vi "V1.2_UI.vi"() -> ()   [LabVIEW 2018]
uses:
  <vilib>/MakerHub/LINX/Private/Type Defs/LINX Ref.ctl
  <vilib>/MakerHub/LINX/Private/Type Defs/Platform.ctl
  <vilib>/MakerHub/LINX/Private/Type Defs/Interface.ctl
  <vilib>/MakerHub/LINX/Private/Device/Type Defs/LINX Device Config.ctl
  <vilib>/MakerHub/LINX/Private/Device/Type Defs/TCP Config.ctl
  <vilib>/MakerHub/LINX/Private/Device/Type Defs/Channels.ctl
  C:/Users/e14user/Documents/LabVIEW software/GitRepo/lib/tiff/LVTiffWriter/BitMiracle.LibTiff.NET.dll
  lib/tiff/LVTiffWriter/BitMiracle.LibTiff.NET.dll
  <vilib>/MakerHub/LINX/Public/Utilities/Open Serial.vi
  lib/Olympus IX BX Series/Olympus IX BX Series.lvlib
  <vilib>/MakerHub/LINX/LMH-LINX.lvlib
  lib/SOLA/LabVIEW 2015 Library (32bit)/LumencorDLL32/LumencorDLL32.lvlib
  lib/ANDOR/Andor SDK/AndorSDK.lvlib
  lib/ANDOR/OwnVIs/AndorOWN.lvlib
  lib/TANGO Stage/TangoOWN.lvlib
  <userlib>/Tango_DLL/Tango_DLL.lvlib
  lib/ARDUINO/VIs/Arduino.lvlib
  lib/Config/Config.lvlib
  lib/tiff/LVTiffWriter/LVTiffWriter.lvlib
  lib/ContinuousLoop/ContinousLoop.lvlib
  <vilib>/vision/NI_Vision_Development_Module.lvlib
  lib/Calib/Calibration.lvlib
  <vilib>/MakerHub/LINX/Private/Device/Device.lvlib
panel:
  out "CalibRemainingTime":dbl caption="Rem. Time" format="%<%H:%M:%S%2u>t"
  in  "CalibRestart":bool
  in  "Calib Feed Cycles":i32=3 caption="Feed Cycles"
  in  "Calib Pump Cycles":i32=10 caption="Pump Cycles"
  in  "AndorHistRange":cluster{"Minimum":sgl, "Maximum":sgl}={"Minimum"=0.0, "Maximum"=65535.0} caption="Range" {"Maximum" min=217 max=912 scale=217.0..912.0; "Minimum" min=217 max=912 scale=217.0..912.0}
  out "ANDORHistMaxValue":dbl
  out "ANDORHistMinValue":dbl
  out "ValveConnSuccess":bool
  in  "ValvePort":refnum<visa-resource-name>="COM7" caption="Valve Controller"
  out "IX81ConnSuccess":bool caption="IX81 Conn Success"
  in  "IX 81 Port":refnum<visa-resource-name>="IX2-UCB"
  out "SOLAConnSuccess":bool
  in  "SOLAPort":refnum<visa-resource-name>="COM5" caption="SOLA COM Port"
  in  "PosListClearLast":bool
  in  "PosListCapture":bool caption="Save Pos"
  out "Program Timing Offset":dbl
  in  "IX81SettingsSave":bool caption="Save Microscope Settings"
  in  "ProgramRun":bool
  out "CalibTiffHandle":refnum<k24> caption="TiffHandle"
  out "CalibInstructions":string="First, capture a blank by adjusting the microscope for a brightfield image of the empty channel. Adjust exposure, objective and filters accordingly. Test it using single images!" caption="Instructions"
  in  "ProgramCreate":bool
  in  "IX81SettingsClear":bool caption="Clear Microscope Settings"
  in  "IX81SettingsAppend":bool caption="Append Current Settings"
  out "CalibImgPath":path caption="Location of Calibration Image File"
  in  "CalibPumpCycleRefreshRatio":dbl=0.01 caption="singlePumpCycleRefreshRatio"
  in  "IX81Settings":i32(listbox) caption="Microscope Settings"
  in  "CalibStart":bool
  out "ProgramProgress":u8(slide) scale=0.0..100.0
  in  "ProgramStop":bool
  out "error out":errorcluster
  out "ProgramXML":string caption="XML"
  out "LINX Resource":T1={"IO"=enum."Remote", "Interface"=enum."TCP", "LINX Device Config"={"Interface"=enum."Serial", "COM Port"="COM13", "TCP Configuration"={"IP Address"="", "Port"=0}, "Device Family"=1, "Device ID"=1, "Device Name"="myRIO-1900", "TCP Ref"=refnum, "Channels"={"DI"=[0, 1, 2, 3, 4, 5, 6, 7, 8, 9, 10, 11, 12, 13, 14, 15, 16, 17, 18, 19, 20, 21, 22, 23, 24, 25, 26, 27, 28, 29, 30, 31, 32, 33, 34, 35, 36, 37, 38, 39, 40, 41, 42, 43, 44, 45, 46], "DO"=[0, 1, 2, 3, 4, 5, 6, 7, 8, 9, 10, 11, 12, 13, 14, 15, 16, 17, 18, 19, 20, 21, 22, 23, 24, 25, 26, 27, 28, 29, 30, 31, 32, 33, 34, 35, 36, 37, 38, 39, 40, 41, 42, 43, 44, 45, 46], "AI"=[0, 1, 2, 3, 4, 5, 6, 7, 8, 9, 10, 11], "AO"=[], "PWM"=[3, 5, 6, 9, 10], "QE"=[], "UART"=[0, 1], "I2C 2"=[0], "SPI"=[0], "CAN"=[], "Servo"=[], "AI Ref (V)"=0.0, "AI Resolution (Bits)"=0, "AO Ref (V)"=0.0, "AO Resolution (Bits)"=0}}}
  out "elements":cluster{"Button":string, "Value":dbl}[](array[cluster])
  out "ANDORAcqErrors":cluster{i32, string}[](array[cluster]) caption="Acqisition Error Array"
  out "ProgramKeysPressed":T7(array[ring]) caption="keys pressed"
  out "TANGOConnError":i32 caption="Tango Connection\n Error"
  in  "PosListSaveXML":bool caption="Save Pos List"
  in  "PosList":i32[](listbox) caption="Position List"
  in  "ValveOpenAll":bool caption="Open all"
  in  "ValveCloseAll":bool caption="Close all"
  in  "C8":bool
  in  "C7":bool
  in  "C6":bool
  in  "C5":bool
  in  "C4":bool
  in  "C3":bool
  in  "C2":bool
  in  "C1":bool
  in  "B8":bool
  in  "B7":bool
  in  "B6":bool
  in  "B5":bool
  in  "B4":bool
  in  "B3":bool
  in  "B2":bool
  in  "B1":bool
  in  "A8":bool
  in  "A7":bool
  in  "A6":bool
  in  "A5":bool
  in  "A4":bool
  in  "A3":bool
  in  "A2":bool
  in  "A1":bool
  in  "ANDORColormap":u16(ring) caption="Colormap" items=["Grey", "Hot"]
  in  "ANDORImgFormat":u16(ring)=6 caption="Format"
  in  "ANDORImgPath":path caption="Path"
  in  "ANDORImgName":string="TestIMG" caption="Image Name"
  in  "ANDORImgSave":bool caption="ANDORSave Image"
  out "SOLA":u32
  out "TANGO":i32
  out "ANDORExposureMeas":sgl caption="Exposure" format="%#_g s"
  out "ANDORAccum":sgl caption="Accum."
  out "ANDORKinetic":sgl caption="Kinetic"
  out "ANDORTemperature":sgl caption="Temperature" format="%.2f °C"
  out "ANDORImage":T8(plugin-control)
  in  "IX81Filter":u16(ring)=6 caption="Filter:" items=["UV ", "CFP", "YFP", "RFP", "Cy5", "GFP", "Bright Field"]
  in  "IX81Prism":u16(ring)=1 caption="Prism" items=["Bi", "Side"]
  in  "IX81Objective":enum16{"x 4", "x 10", "x 20", "x 40", "x 100"}(ring) caption="Objective"
  in  "IX81Focus":dbl caption="Focus [µm]" format="%.3f"
  out "IX81LimitTop":dbl caption="Upper Limit"
  out "IX81LimitBottom":dbl caption="Lower Limit"
  in  "IX81Intensity":dbl(slide) caption="Intensity [%]" scale=0.0..100.0 scale format="%.1f"
  in  "ANDORExposure":sgl=50.0 caption="Exposure" format="%#_g ms"
  in  "ANDORLive":bool
  in  "ANDORImgSingle":bool
  in  "TANGODown":bool
  in  "TANGOLeft":bool caption="Left"
  in  "TANGOUp":bool
  in  "TANGORight":bool
  in  "ProgramSingleMultiring":bool=TRUE caption="Which chip are you using?"
  in  "ValveFeedRingAll":bool caption="Actuate all Rings at once?"
  in  "ValveFlushReagent":u16 caption="Flush\nReagent"
  in  "ValveFlushOn":bool caption="Flush"
  in  "ValvePumpCycles":dbl=10.0 caption="Pump Cycles"
  in  "ValvePumpFrequency":dbl=10.0 caption="Frequency" format="%#_3f"
  in  "ValvePumpOn":bool caption="Pump On"
  in  "ValveFeedOn":bool caption="Feed On"
  in  "ValveFeedCycles":i32=10 caption="Feed Cycles"
  in  "ValveFeedReagent":u16=2 caption="Feed\nReagent"
  in  "ValveFeedRing":u16 caption="Ring"
  in  "TANGOCalibrate":bool caption="Calibrate"
  out "TANGOyLimits":dbl[](array[numeric]) caption="Y Limits [µm]" format="%#_12f"
  out "TANGOxLimits":dbl[](array[numeric]) caption="X Limits [µm]" format="%#_10f"
  in  "TANGOStep":dbl=100.0 caption="Step Width [µm]" min=0.0 format="%#_6f"
  out "TANGOPosition":dbl[](array[numeric]) caption="Position [µm]" format="%#_12f"
  out "TANGOConnSuccess":bool
  in  "TANGOPort":refnum<visa-resource-name>="COM4" caption="TANGO COM Port"
  out "ProgramStatusInfo":string caption="String"
  # "Calibration of a Microfluidic Pump"
  # "Execute Continuous Progam"
  # "Error Messages"
  # "More information below"
  # "Various Error and Status Messages"
  # "Position List"
  # "Manual Valves"
  # "Save Image"
  # "OneRing"
  # "Multiring"
  # "Microfluidics"
  # "Valve Functions"
  # "min"
  # "max"
  # "min"
  # "max"
  # "X"
  # "Y"
  # "Stage"
  # "Initialization"
  # "Microscope"
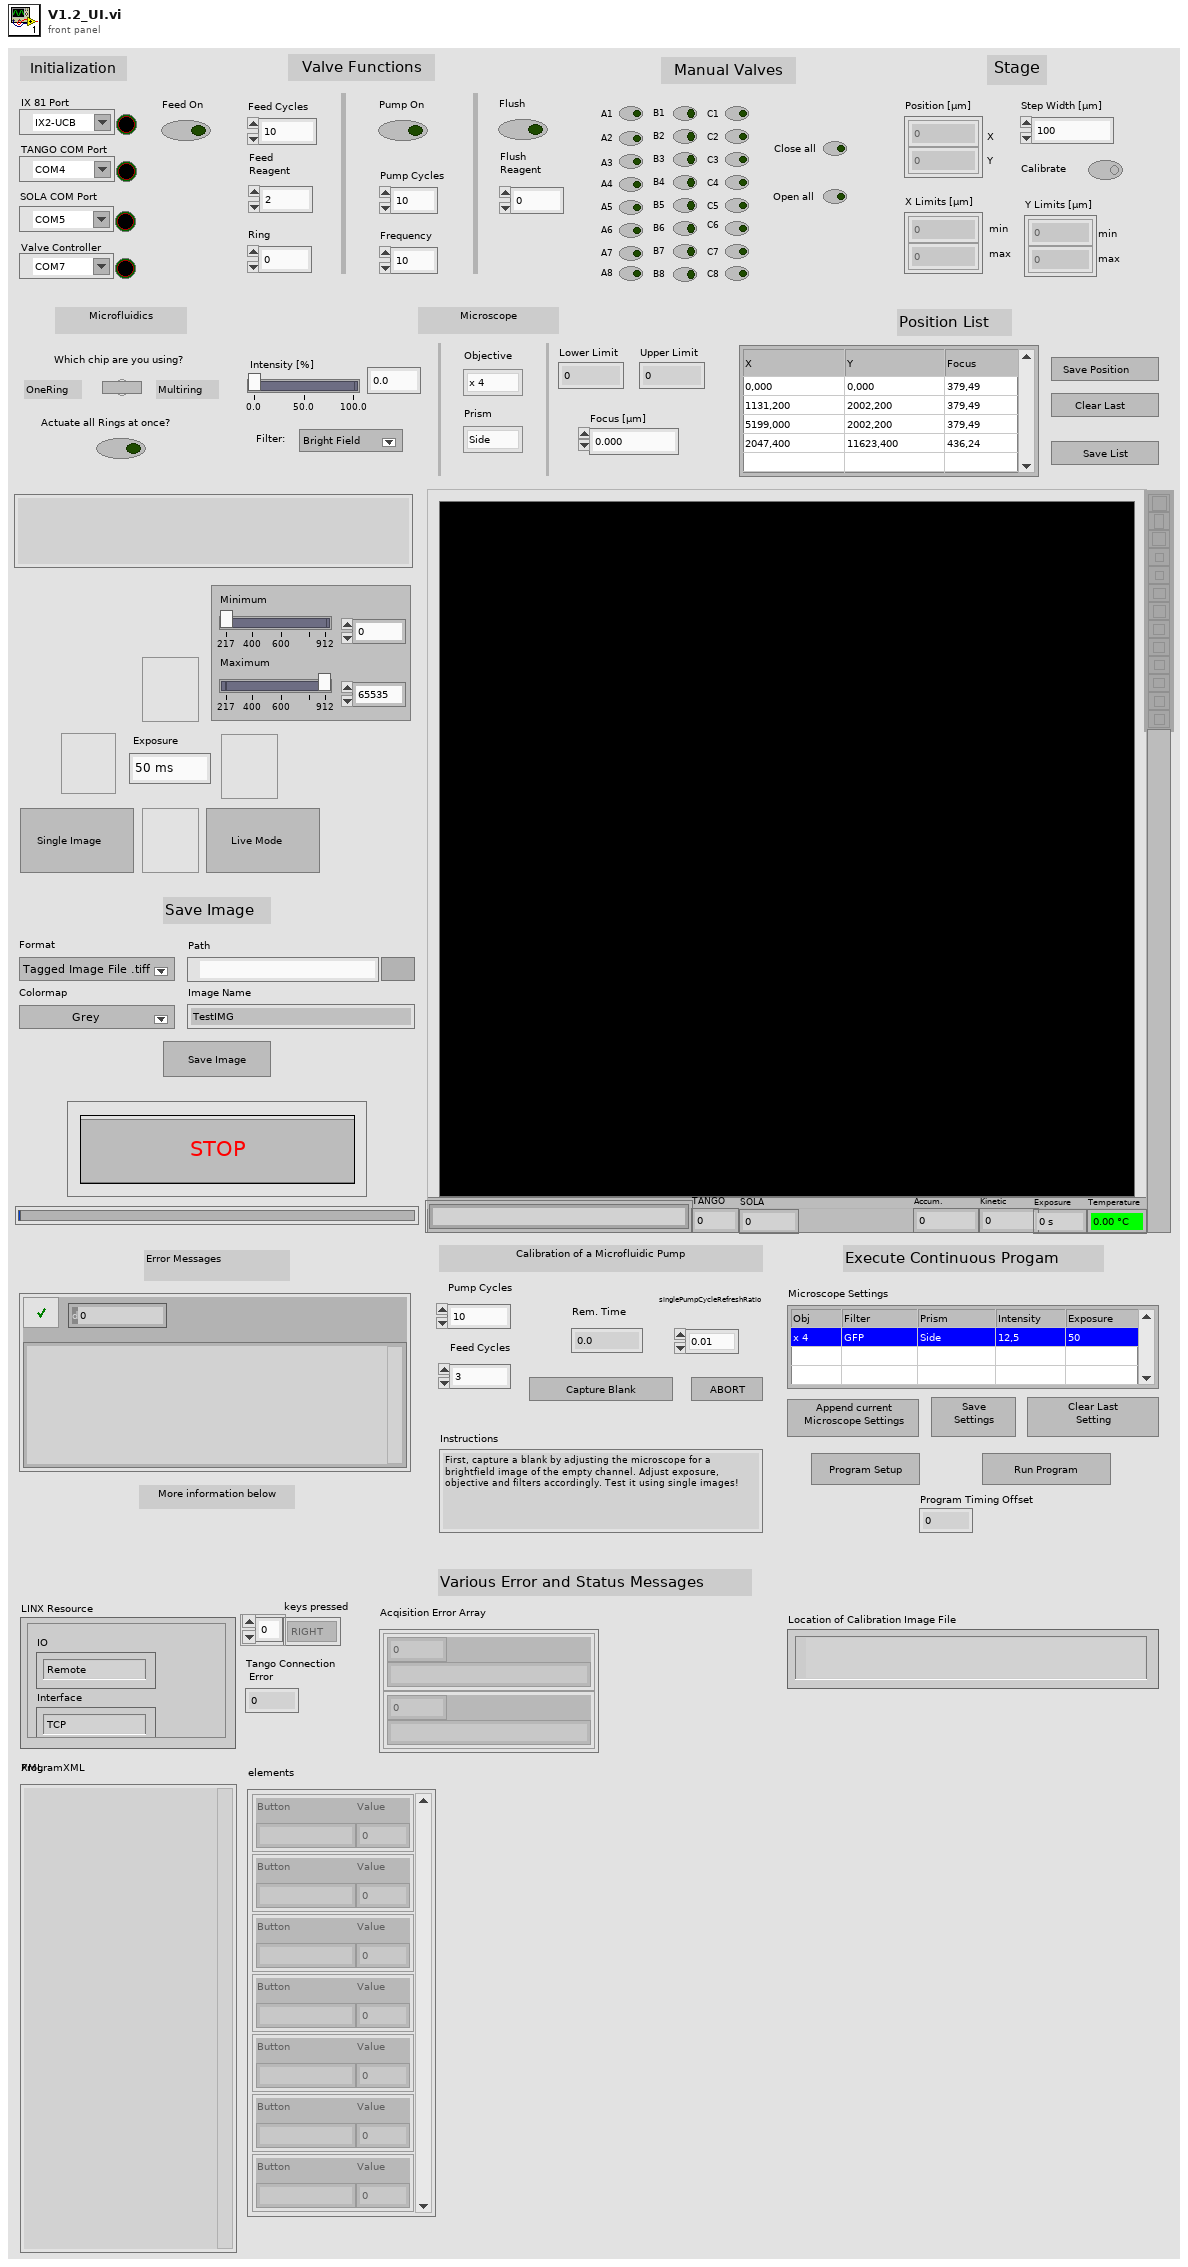
[diagram p1: front panel]
types:
  T1 = typedef "LMH-LINX.lvlib/LINX Ref.ctl" = cluster{"IO":T2, "Interface":T3, "LINX Device Config":T4}
  T2 = typedef "LMH-LINX.lvlib/Platform.ctl" = enum16{"Remote", "Local"}
  T3 = typedef "LMH-LINX.lvlib/Interface.ctl" = enum16{"Serial", "TCP"}
  T4 = typedef "LMH-LINX.lvlib/Device.lvlib/LINX Device Config.ctl" = cluster{"Interface":T3, "COM Port":refnum<visa-resource-name>, "TCP Configuration":T5, "Device Family":u8, "Device ID":u8, "Device Name":string, "TCP Ref":refnum<k5>, "Channels":T6}
  T5 = typedef "LMH-LINX.lvlib/Device.lvlib/TCP Config.ctl" = cluster{"IP Address":string, "Port":u16}
  T6 = typedef "LMH-LINX.lvlib/Channels.ctl" = cluster{"DI":u8[], "DO":u8[], "AI":u8[], "AO":u8[], "PWM":u8[], "QE":u8[], "UART":u8[], "I2C 2":u8[], "SPI":u8[], "CAN":u8[], "Servo":u8[], "AI Ref (V)":dbl, "AI Resolution (Bits)":u8, "AO Ref (V)":dbl, "AO Resolution (Bits)":u8}
  T7 = enum16{"0", "1", "2", "3", "4", "5", "6", "7", "8", "9", "A", "B", "C", "D", "E", "F", "G", "H", "I", "J", "K", "L", "M", "N", "O", "P", "Q", "R", "S", "T", "U", "V", "W", "X", "Y", "Z", "F1", "F2", "F3", "F4", "F5", "F6", "F7", "F8", "F9", "F10", "F11", "F12", "F13", "F14", "F15", "ADD", "BACK", "BACKSLASH", "CAPITAL", "COMMA", "DECIMAL", "DELETE", "DIVIDE", "DOWN", "END", "EQUALS", "ESCAPE", "GRAVE (`)", "HOME", "INSERT", "LBRACKET", "LCONTROL", "LEFT", "L ALT", "LSHIFT", "LWIN", "MINUS", "MULTIPLY", "NEXT", "NUMLOCK", "NUMPAD_0", "NUMPAD_1", "NUMPAD_2", "NUMPAD_3", "NUMPAD_4", "NUMPAD_5", "NUMPAD_6", "NUMPAD_7", "NUMPAD_8", "NUMPAD_9", "PAUSE", "PERIOD", "PRIOR (PG UP)", "RBRACKET", "RCONTROL", "RETURN", "RIGHT", "R ALT", "RSHIFT", "RWIN", "SCROLL", "SEMICOLON", "SLASH", "SPACE", "SUBTRACT", "TAB", "UP", "ENTER (num pad)", "' (quote)"}[]
  T8 = typedef "IMAQ Image.ctl" = refnum<image>
  T9 = enum8{"Enabled", "Disabled", "Disabled and Grayed Out"}
  T10 = enum32{"Linear", "Log", "Exp", "Square", "Square root", "Power X", "Power 1/X"}
  T11 = enum16{"open", "replace", "create", "open or create", "replace or create", "replace or create with confirmation"}
  T12 = typedef "Image Type" = u32
  T13 = cluster{"histogram":u32[], "Minimal Value":sgl, "Maximal Value":sgl, "Starting Value":sgl, "Interval Width":sgl, "Mean Value":sgl, "Standard  Variation":sgl, "Area (pixels)":i32}
  T14 = cluster{string, "NewVal":enum16{"x 4", "x 10", "x 20", "x 40", "x 100"}}
  T15 = cluster{"Objective":i32, "Filter":string, "Prism":string, "Intensity":dbl, "Exposure":i32}[]
  T16 = cluster{"Step Name":string, "Time":dbl, "Param 1":dbl, "Param 2":i32}
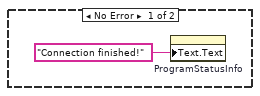
[diagram p2: hidden frame]
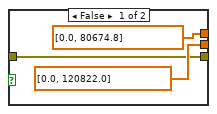
[diagram p3: hidden frame]
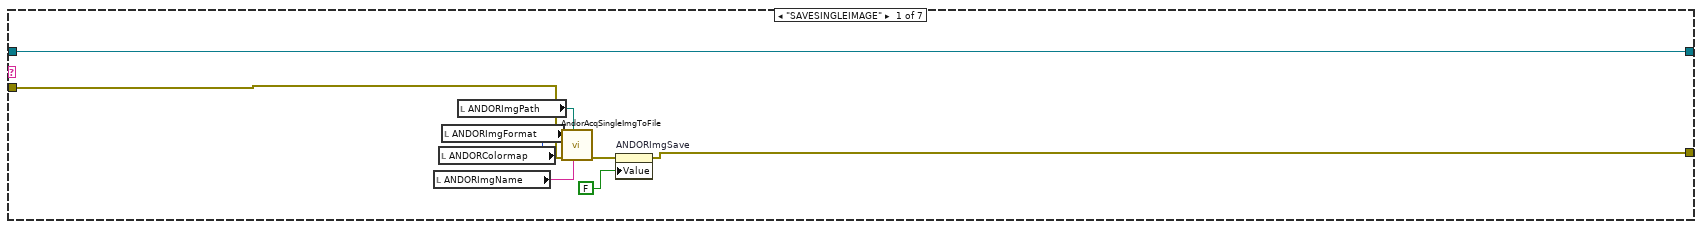
[diagram p4: hidden frame]
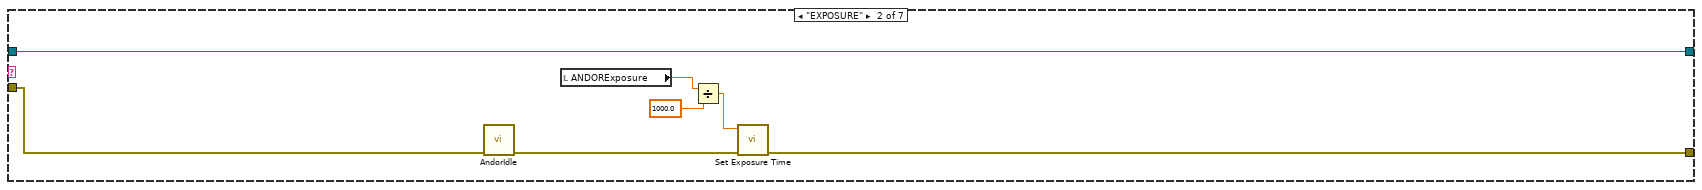
[diagram p5: hidden frame]
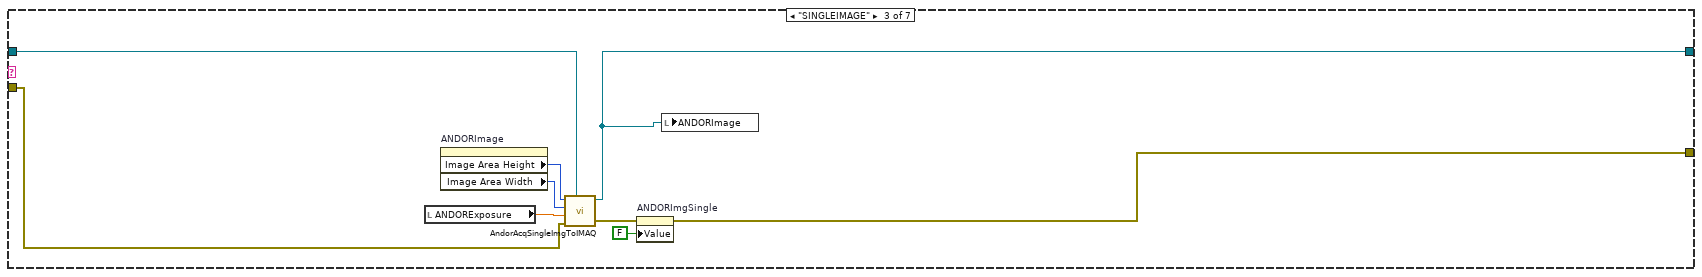
[diagram p6: hidden frame]
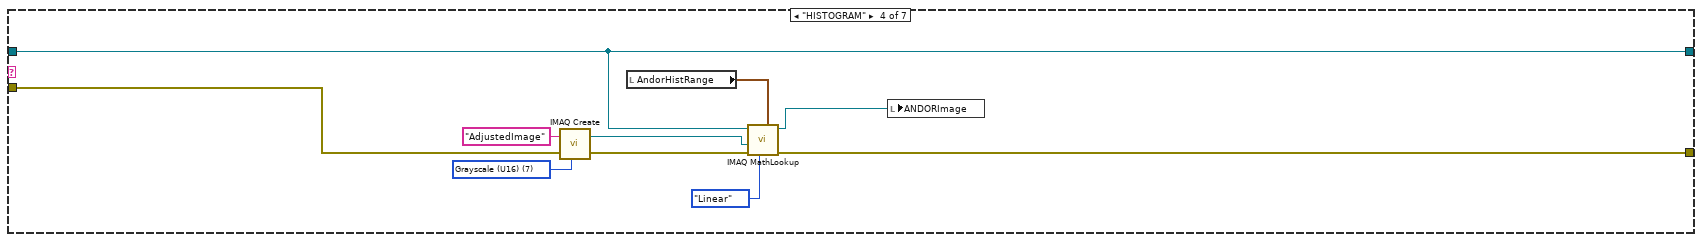
[diagram p7: hidden frame]
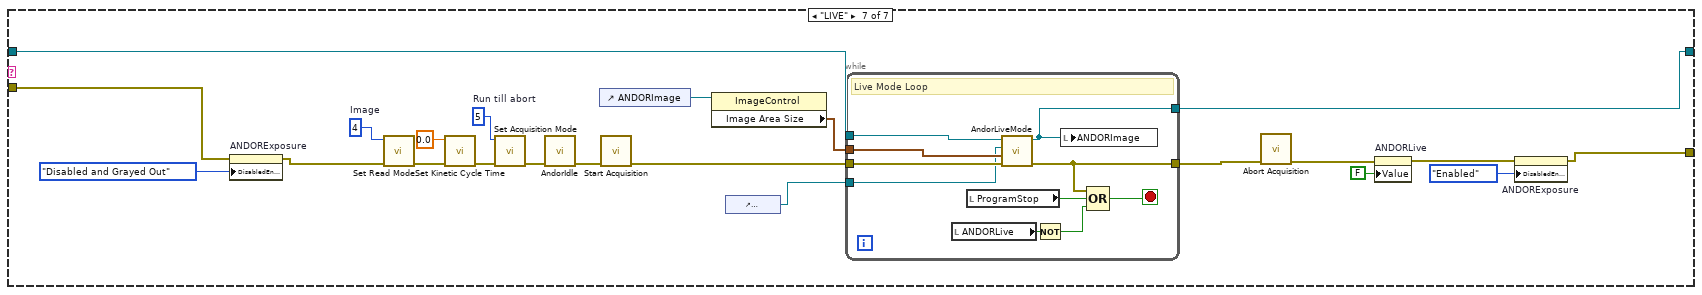
[diagram p9: hidden frame]
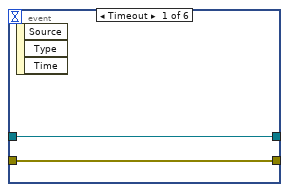
[diagram p10: hidden frame]
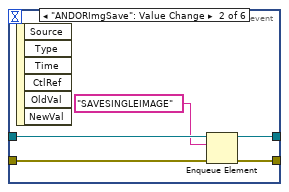
[diagram p11: hidden frame]
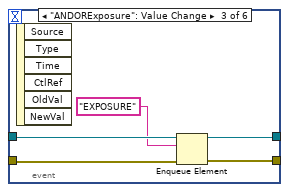
[diagram p12: hidden frame]
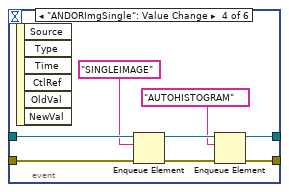
[diagram p13: hidden frame]
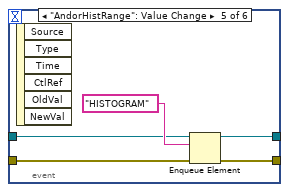
[diagram p14: hidden frame]
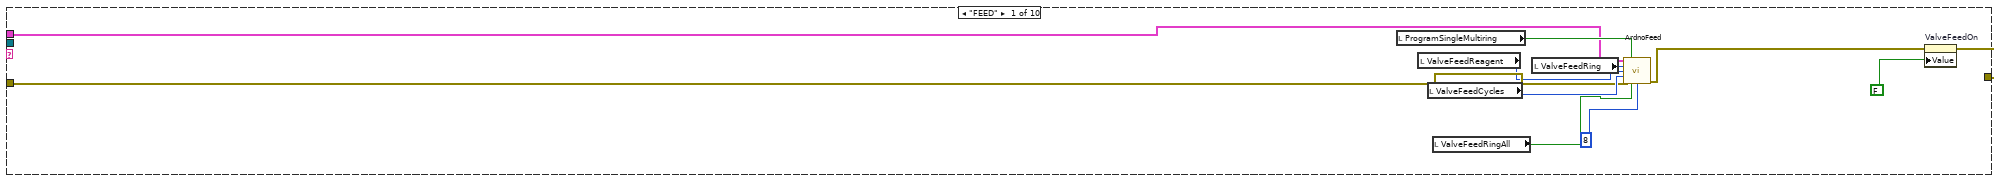
[diagram p16: hidden frame]
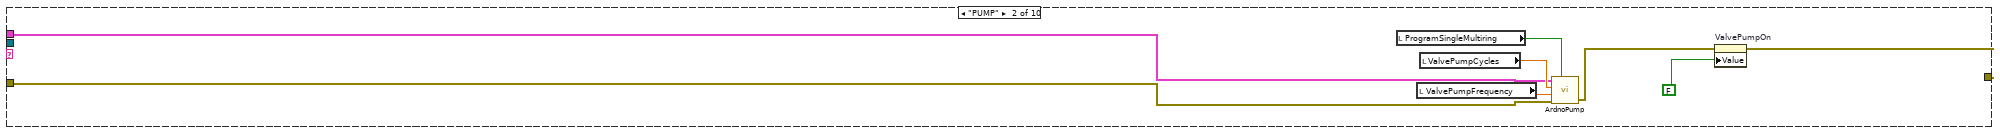
[diagram p17: hidden frame]
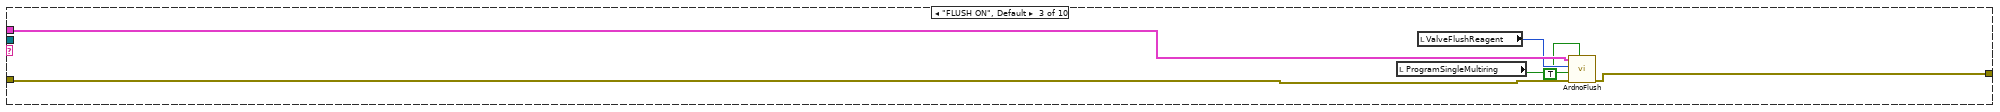
[diagram p18: hidden frame]
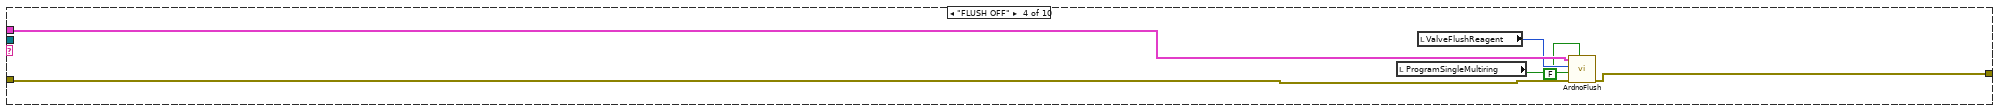
[diagram p19: hidden frame]
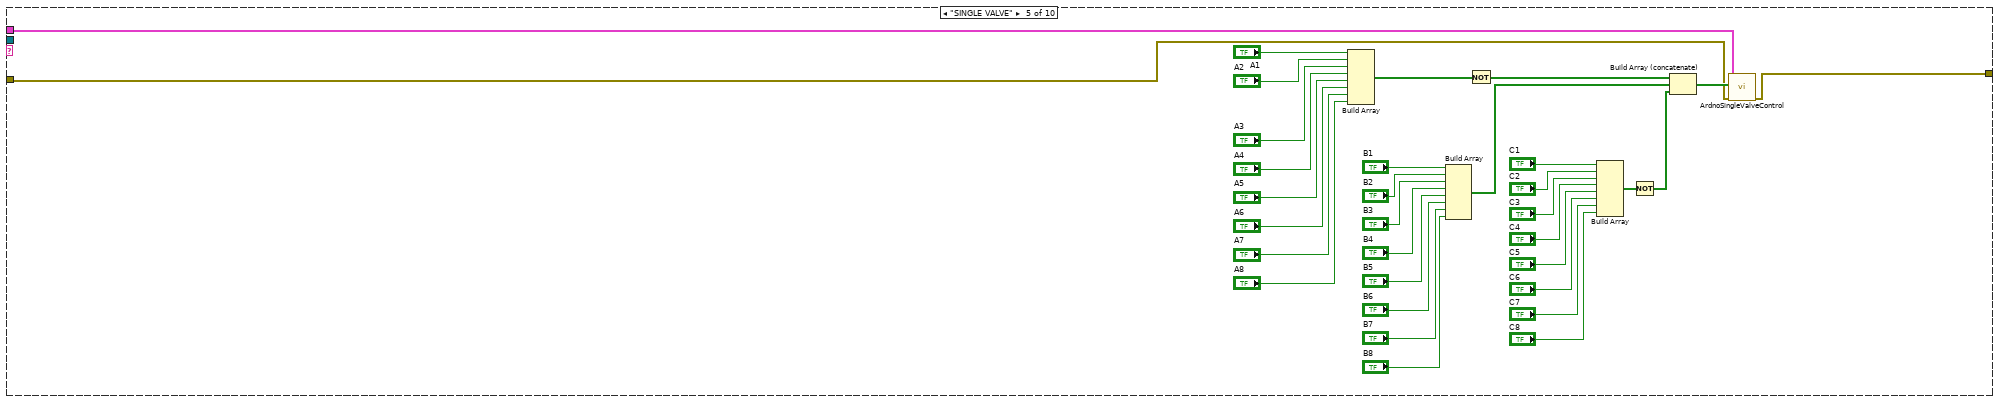
[diagram p20: hidden frame]
diagram:
  n1 = flat-sequence {
    tunnel: [w32] -> w9
    tunnel: [w31] -> w8
    tunnel: [w30] -> w7
    tunnel: [w29] -> w6
    tunnel: [w28] -> w5
    tunnel: [w80] -> w19
    tunnel: w9 -> [w73]
    tunnel: w8 -> [w72]
    tunnel: w7 -> [w71]
    tunnel: w6 -> [w65]
    tunnel: w5 -> [w70]
    tunnel: [w69] -> w4
    tunnel: [w68] -> w3
    tunnel: [w64] -> w2
    tunnel: [w67] -> w1
    tunnel: [w109] -> w20
    tunnel: w19 -> [w110]
    tunnel: w4 -> [w108]
    tunnel: w3 -> [w107]
    tunnel: w2 -> [w106]
    tunnel: w1 -> [w105]
    tunnel: w20 -> [w1609]
    tunnel: [w1603] -> w12
    frame #0 {
      w21 = cluster{u32, u32}[] [{16711680, 0}, {65280, 0}, {6710886, 0}, {6710886, 0}] ("Colors [4]")
      # "Connection String"
      n2 = local write "ProgramStatusInfo"("Connecting..." ("Info")) -> ()
      n3 = property on="CalibStart" class="Bool (strict)"("BoolText.Text"="Capture Blank" ("Boolean Text.Text")) -> ()  [unwired: 2 in, 2 out]
      n4 = property on="Pane" class="Pane"() -> ("Controls[]"=w23:refnum<vi>[])  [unwired: 2 in, 2 out]
      n5 = for {
        tunnel: w23 -> [w27] mode=indexing
        tunnel: T9."Enabled" ("Disabled") -> [w26]
        n6 = property class="Ctl"(reference=w27, "DisabledEnum"=w26) -> ()  [unwired: 1 in, 2 out]
      }
      n7 = property on="IX81ConnSuccess" class="Bool (strict)"("Colors [4]"=w21) -> ()  [unwired: 2 in, 2 out]
      n8 = property on="TANGOConnSuccess" class="Bool (strict)"("Colors [4]"=w21) -> ()  [unwired: 2 in, 2 out]
      n9 = property on="SOLAConnSuccess" class="Bool (strict)"("Colors [4]"=w21) -> ()  [unwired: 2 in, 2 out]
      n10 = property on="ValveConnSuccess" class="Bool (strict)"("Colors [4]"=w21) -> ()  [unwired: 2 in, 2 out]
    }
    frame #1 {
      w55 = 2  # Device Number (1: Condensor, Objective Lamp,Shutter 2: Z-Motion, Autofocus)
      w58 = 1  # Device Number (1: Condensor, Objective Lamp,Shutter 2: Z-Motion, Autofocus)
      # "Establishing Connections To All Devices"
      n11 = property on="SOLAPort" class="VISAName"() -> ("Text.Text"=w42:string)  [unwired: 2 in, 2 out]
      n12 = Scan From String(format string="COM%d", input string=w42) -> (output 1=w51:i32)  [unwired: 3 in, 3 out]
      n13 = local read "TANGOPort"() -> (w45:refnum<visa-resource-name>)
      n14 = local read "ValvePort"() -> (w53:refnum<visa-resource-name>)
      n15 = Decrement(x=w51) -> (x-1=w50:i32)
      n16 = local read "IX 81 Port"() -> (w54:refnum<visa-resource-name>)
      n17 = call-poly <vilib>:"Open.vi"("Serial Port"=w53) -> ("Error Out"=w29:errorcluster, "LINX Resource"=→"LINX Resource":T1)  [unwired: 8 in, 1 out]
      n18 = call "lm Init.vi"("LETypeStr"="SOLA", "ComPort"=w50) -> ("error out"=w30:errorcluster, "LETypeStr out"=w41:string, "function return"=→"SOLA":u32)  [unwired: 7 in]
      n19 = call "Initialize.vi"("VISA Resource Name"=w54) -> ("VISA Resource Name Out"=w59:refnum<visa-resource-name>, "error out"=w60:errorcluster)  [unwired: 13 in]
      n20 = call "Initialize.vi"("dir"="C:\\Users\\e14user\\Documents\\LabVIEW software\\GitRepo\\lib\\ANDOR\\Libraries") -> ("error out"=w31:errorcluster)  [unwired: 8 in, 2 out]
      n21 = call "TangoConnect.vi"("Tango Com"=w45) -> ("error out"=w32:errorcluster, "success"=w43:bool, "plLSID out"=→"TANGO":i32)  [unwired: 7 in, 1 out]
      n22 = Unbundle By Name(w30) -> ("status"=w39:bool)
      n23 = Unbundle By Name(w29) -> ("status"=w35:bool)
      n24 = call "Login Device.vi"("error in (no error)"=w60, "Device Number (1)"=w58, "VISA Resource Name"=w59) -> ("error out"=w56:errorcluster, "VISA Resource Name Out"=w57:refnum<visa-resource-name>)  [unwired: 7 in]
      n25 = Empty String/Path?(string/path=w41) -> (empty?=w40:bool)
      n26 = local write "TANGOConnSuccess"(w43) -> ()
      n27 = Not(x=w35) -> (.not. x?=w34:bool)
      n28 = Not Or(1:w39, 2:w40) -> (0:w38:bool)
      n29 = call "Login Device.vi"("error in (no error)"=w56, "Device Number (1)"=w55, "VISA Resource Name"=w57) -> ("error out"=w28:errorcluster)  [unwired: 7 in, 1 out]
      n30 = local write "ValveConnSuccess"(w34) -> ()
      n31 = local write "SOLAConnSuccess"(w38) -> ()
      n32 = Unbundle By Name(w28) -> ("status"=w37:bool)
      n33 = Not(x=w37) -> (.not. x?=w33:bool)
      n34 = local write "IX81ConnSuccess"(w33) -> ()
      n35 = Merge Errors(w28, w29, w30, w32, w31) -> (w47:errorcluster)
      n36 = case shown="Error" w47 {
        frame No Error {
          n37 = property on="ProgramStatusInfo" class="Str"("Text.Text"="Connection finished!") -> ()  [unwired: 2 in, 2 out]
        }
        frame Error {
          n38 = property on="ProgramStatusInfo" class="Str"("Text.Text"="Connection did not work!\nTry restarting the respective device.") -> ()  [unwired: 2 in, 2 out]
        }
      }
    }
    frame #2 {
      # "Initializing Devices With (Config File)"
      n39 = local read "LINX Resource"() -> (w66:T1)
      n40 = local read "IX 81 Port"() -> (w94:refnum<visa-resource-name>)
      n41 = local read "ANDORExposure"() -> (w85:sgl)
      n42 = local read "TANGOCalibrate"() -> (w89:bool)
      n43 = local write "IX81LimitTop"(3000000.0 ("default (0 I32)")) -> ()
      n44 = local write "IX81LimitBottom"(10.0 ("Upper Limit")) -> ()
      n45 = call "AndorInitCamera.vi"("error in (no error)"=w72, "Exposure"=w85) -> ("error out"=w69:errorcluster, "accumulate out"=w82:sgl, "exposure out"=w83:sgl, "temperature out"=w86:sgl, "kinetic out"=w84:sgl)  [unwired: 5 in]
      n46 = call "lm Color Enable.vi"("error in (no error)"=w71, "str_State"="ON", "str_Color"="WHITE") -> ("error out"=w75:errorcluster, "str_Color out"=w76:string)  [unwired: 6 in, 1 out]
      n47 = call "OlympusInitialize.vi"("error in (no error)"=w70, "IX81 in"=w94) -> ("error out"=w67:errorcluster, "Objective"=w92:i32, "Focus Position"=w81:dbl, "Prism Position (0: Bi)"=w78:enum16{"Bi", "Side"}, "Filter"=w93:i32, "Intensity [%]"=w79:dbl)  [unwired: 4 in]
      n48 = case shown="True" w89 {
        tunnel: [w97 w104] -> w68
        tunnel: w73 -> [w97 w100]
        tunnel: [dbl[] [0.0, 80674.8] ("Y Limits") w103] -> w87
        tunnel: [dbl[] [0.0, 120822.0] ("X Limits") w102] -> w88
        frame False {
        }
        frame True {
          n49 = local read "TANGO"() -> (w101:i32)
          n50 = call "TangoCalibrate.vi"("error in (no error)"=w100, "plLSID in"=w101) -> ("error out"=w104:errorcluster, "X Limits"=w102:dbl[], "Y Limits"=w103:dbl[])  [unwired: 7 in]
        }
      }
      n51 = call "ArdnoAllValvesOpened.vi"("Single/\nMultiring?"=TRUE ("Single/\nMultiring?"), "error in (no error)"=w65, "LINX Resource"=w66) -> ("error out"=w64:errorcluster)  [unwired: 7 in, 1 out]
      n52 = local write "ANDORKinetic"(w84) -> ()
      n53 = local write "ANDORTemperature"(w86) -> ()
      n54 = local write "ANDORExposureMeas"(w83) -> ()
      n55 = local write "ANDORAccum"(w82) -> ()
      n56 = call "lm Color Level.vi"("error in (no error)"=w75, "str_Level"="0", "str_Color"=w76) -> ("error out"=w74:errorcluster)  [unwired: 6 in, 2 out]
      n57 = local write "TANGOyLimits"(w87) -> ()
      n58 = local write "TANGOxLimits"(w88) -> ()
      n59 = local write "IX81Intensity"(w79) -> ()
      n60 = local write "IX81Prism"(w78) -> ()
      n61 = local write "IX81Focus"(w81) -> ()
      n62 = local write "IX81Objective"(w92) -> ()
      n63 = local write "IX81Filter"(w93) -> ()
      n64 = Merge Errors(w67, w64, w74, w68, w69) -> (w80:errorcluster)
    }
    frame #3 {
      n65 = while {
        shift-right: [w117] -> w109
        shift-left: w110 -> [w116]
        tunnel: w108 -> [w114]
        tunnel: w107 -> [w113]
        tunnel: w106 -> [w112]
        tunnel: w105 -> [w111]
        stop <- w115 stop-if-true
        n66 = stacked-sequence {
          tunnel: [w122 _] -> w117
          tunnel: w116 -> [_ _]
          tunnel: w114 -> [w121 _]
          tunnel: w113 -> [w120 _]
          tunnel: w112 -> [w119 _]
          tunnel: w111 -> [w118 _]
          frame #0 {
            n67 = while {
              tunnel: w120 -> [w151]
              tunnel: w119 -> [w150]
              tunnel: w118 -> [w149]
              shift-right: [w123] -> w122
              shift-left: w121 -> [w152]
              stop <- w126 stop-if-true
              w136 = 1122  # Clear Queue Invalid Error
              w162 = T12 7 items=["Grayscale (U8)", "Grayscale (I16)", "Grayscale (SGL)", "Complex (CSG)", "RGB (U32)", "HSL (U32)", "RGB (U64)", "Grayscale (U16)"] ("Image Type")
              w194 = ""  # Button
              n68 = call "IMAQ Create"("Image Name"="RawImage", "Image Type"=w162) -> ("New Image"=w163:T8, "error out"=w145:errorcluster)  [unwired: 3 in]
              n69 = local read "TANGO"() -> (w205:i32)
              n70 = local read "LINX Resource"() -> (w201:T1)
              n71 = Obtain Queue(name (unnamed)="CameraQueue", element data type="", error in (no error)=w152) -> (queue out=w185:refnum<queue>, error out=w184:errorcluster)  [unwired: 2 in, 1 out]
              n72 = Obtain Queue(name (unnamed)="StageCTRL", element data type="" ("Button"), error in (no error)=w151) -> (queue out=w197:refnum<queue>, error out=w177:errorcluster)  [unwired: 2 in, 1 out]
              n73 = local read "IX 81 Port"() -> (w167:refnum<visa-resource-name>)
              n74 = Obtain Queue(name (unnamed)="FluidCTRL", element data type=w194, error in (no error)=w150) -> (queue out=w200:refnum<queue>, error out=w199:errorcluster)  [unwired: 2 in, 1 out]
              n75 = Obtain Queue(name (unnamed)="MicroscopeCTRL", element data type=cluster{"Button":string, "Value":dbl} {"Button"="", "Value"=0.0}, error in (no error)=w149) -> (queue out=w196:refnum<queue>, error out=w148:errorcluster)  [unwired: 2 in, 1 out]
              n76 = Merge Errors(w145, w184) -> (w146:errorcluster)
              n77 = while {
                tunnel: 5 -> [w297]
                tunnel: w185 -> [w292]
                tunnel: [w290] -> w156
                tunnel: w184 -> [w291]
                tunnel: [w289] -> w154
                stop <- w294 stop-if-true
                # "ANDOR CAMERA MEssage Loop"
                n78 = event shown="[5] \"ANDORLive\": Value Change" {
                  selector: _ -> [_ _ _ _ _ _]
                  dyn-events: _ -> [_ _ _ _ _ _]
                  timeout: w297 -> [_ _ _ _ _ _]
                  tunnel: w292 -> [w299 w304 w309 w317 w321 w329]
                  tunnel: w291 -> [w298 w303 w308 w316 w320 w330]
                  tunnel: [w298 w300 w306 w311 w319 w323] -> w289
                  tunnel: [w299 w301 w307 w313 w318 w324] -> w290
                  event Timeout {
                    n79 = event-data() -> ()  [unwired: 1 in, 3 out]
                  }
                  event "ANDORImgSave": Value Change {
                    n80 = event-data() -> ()  [unwired: 1 in, 6 out]
                    n81 = Enqueue Element(queue=w304, element="SAVESINGLEIMAGE", error in (no error)=w303) -> (queue out=w301:refnum<queue>, error out=w300:errorcluster)  [unwired: 1 in, 1 out]
                  }
                  event "ANDORExposure": Value Change {
                    n82 = event-data() -> ()  [unwired: 1 in, 6 out]
                    n83 = Enqueue Element(queue=w309, element="EXPOSURE", error in (no error)=w308) -> (queue out=w307:refnum<queue>, error out=w306:errorcluster)  [unwired: 1 in, 1 out]
                  }
                  event "ANDORImgSingle": Value Change {
                    n84 = event-data() -> ()  [unwired: 1 in, 6 out]
                    n85 = Enqueue Element(queue=w317, element="SINGLEIMAGE", error in (no error)=w316) -> (queue out=w314:refnum<queue>, error out=w312:errorcluster)  [unwired: 1 in, 1 out]
                    n86 = Enqueue Element(queue=w314, element="AUTOHISTOGRAM", error in (no error)=w312) -> (queue out=w313:refnum<queue>, error out=w311:errorcluster)  [unwired: 1 in, 1 out]
                  }
                  event "AndorHistRange": Value Change {
                    n87 = event-data() -> ()  [unwired: 1 in, 6 out]
                    n88 = Enqueue Element(queue=w321, element="HISTOGRAM", error in (no error)=w320) -> (queue out=w318:refnum<queue>, error out=w319:errorcluster)  [unwired: 1 in, 1 out]
                  }
                  event "ANDORLive": Value Change {
                    n89 = event-data() -> ("NewVal"=w328:bool)  [unwired: 1 in, 5 out]
                    n90 = case shown="True" w328 {
                      tunnel: w329 -> [w332 w337]
                      tunnel: w330 -> [w331 w335]
                      tunnel: [w332 w334] -> w326
                      tunnel: [w331 w333] -> w325
                      frame False {
                      }
                      frame True {
                        n91 = Enqueue Element(queue=w337, element="LIVE", error in (no error)=w335) -> (queue out=w334:refnum<queue>, error out=w333:errorcluster)  [unwired: 1 in, 1 out]
                      }
                    }
                    n92 = Enqueue Element(queue=w326, element="AUTOHISTOGRAM", error in (no error)=w325) -> (queue out=w324:refnum<queue>, error out=w323:errorcluster)  [unwired: 1 in, 1 out]
                  }
                }
                n93 = local read "ProgramCreate"() -> (w296:bool)
                n94 = local read "ProgramStop"() -> (w295:bool)
                n95 = local read "ProgramRun"() -> (w293:bool)
                n96 = Compound Arithmetic op=OR(w289, w295, w296, w293) -> (w294:bool)
              }
              n97 = while {
                tunnel: 3000 -> [w1138]
                tunnel: w152 -> [w1140]
                tunnel: [w1139] -> w178
                stop <- w1144 stop-if-true
                # "Measure CCD-Sensor Temp every 3s"
                n98 = event shown="[0] Timeout" {
                  selector: _ -> [_]
                  dyn-events: _ -> [_]
                  timeout: w1138 -> [_]
                  tunnel: [w1145] -> w1139
                  tunnel: w1140 -> [w1150]
                  event Timeout {
                    n99 = event-data() -> ()  [unwired: 1 in, 3 out]
                    n100 = call "AndorIdle.vi"("error in (no error)"=w1150) -> ("error out"=w1151:errorcluster)  [unwired: 9 in, 1 out]
                    n101 = call "Get Temperature F.vi"("error in (no error)"=w1151) -> ("error out"=w1147:errorcluster, "temperature out"=w1146:sgl)  [unwired: 8 in, 1 out]
                    n102 = Less?(x=w1146, y=sgl -60.0) -> (x < y?=w1148:bool)
                    n103 = case shown="True" w1148 {
                      tunnel: w1147 -> [w1153 w1157]
                      tunnel: w1146 -> [w1154 w1158]
                      tunnel: [w1152 w1156] -> w1145
                      frame False {
                        n104 = property on="ANDORTemperature" class="DigNum (strict)"(error in=w1153, "Value"=w1154, "NumText.BGColor"=u32 16711680 ("Numeric Text.Text Colors:BG Color")) -> (error out=w1152:errorcluster)  [unwired: 1 in, 1 out]
                      }
                      frame True {
                        n105 = property on="ANDORTemperature" class="DigNum (strict)"(error in=w1157, "Value"=w1158, "NumText.BGColor"=u32 65280 ("Numeric Text.Text Colors:BG Color")) -> (error out=w1156:errorcluster)  [unwired: 1 in, 1 out]
                      }
                    }
                  }
                }
                n106 = local read "ProgramCreate"() -> (w1143:bool)
                n107 = local read "ProgramRun"() -> (w1142:bool)
                n108 = local read "ProgramStop"() -> (w1141:bool)
                n109 = Compound Arithmetic op=OR(w1139, w1141, w1143, w1142) -> (w1144:bool)
              }
              n110 = while {
                tunnel: w197 -> [w712]
                tunnel: w205 -> [w707]
                tunnel: w177 -> [w711]
                tunnel: [w703] -> w133
                stop <- w703 stop-if-true
                # "TANGO Stage Execution Loop"
                n111 = Dequeue Element(queue=w712, error in (no error)=w711) -> (element=w705:string, error out=w706:errorcluster)  [unwired: 1 in, 2 out]
                n112 = Wait (ms)(milliseconds to wait=u32 50) -> ()  [unwired: 1 out]
                n113 = call <vilib>:"Space Constant.vi"() -> ("String"=w710:string)
                n114 = Match Pattern(string=w705, regular expression=w710) -> (before substring=w709:string, after substring=w708:string)  [unwired: 1 in, 2 out]
                n115 = case shown="\"EXPORT\"" w709 {
                  tunnel: w708 -> [w716 w734 w752 w774 _ _ w827 _ _]
                  tunnel: w707 -> [w715 w733 w751 w773 w811 _ w826 _ w840]
                  tunnel: w706 -> [w714 w732 w750 w772 w805 w816 w825 w832 w841]
                  tunnel: [w713 w731 w749 w771 w789 w812 w823 w830 w835] -> w703
                  frame "DOWN", Default {
                    n116 = case shown="\"RELEASED\", Default" w716 {
                      tunnel: w714 -> [w717 w730]
                      tunnel: [w717 w729] -> w713
                      tunnel: w715 -> [_ w721]
                      frame "RELEASED", Default {
                      }
                      frame "PRESSED" {
                        w718 = 0.0 ("bWait")
                        n117 = local read "TANGOStep"() -> (w720:dbl)
                        n118 = Multiply(x=1.0, y=w720) -> (x*y=w722:dbl)
                        n119 = call <userlib>:"LSX Move Rel.vi"("bWait"=w718, "dA"=w718, "dZ"=w718, "error in (no error)"=w730, "dY"=w722, "dX"=w718, "lLSID"=w721) -> ("error out"=w724:errorcluster)  [unwired: 3 in, 1 out]
                        n120 = call <userlib>:"LSX Get Pos.vi"("lLSID"=w721, "error in (no error)"=w724) -> ("pdA out"=w725:dbl, "pdX out"=w728:dbl, "pdY out"=w727:dbl, "pdZ out"=w726:dbl, "error out"=w729:errorcluster)  [unwired: 8 in, 1 out]
                        n121 = Build Array(w728, w727, w726, w725) -> (w719:dbl[])
                        n122 = local write "TANGOPosition"(w719) -> ()
                      }
                    }
                  }
                  frame "UP" {
                    n123 = case shown="\"RELEASED\", Default" w734 {
                      tunnel: w732 -> [w735 w748]
                      tunnel: [w735 w747] -> w731
                      tunnel: w733 -> [_ w739]
                      frame "RELEASED", Default {
                      }
                      frame "PRESSED" {
                        w736 = 0.0 ("dY")
                        n124 = local read "TANGOStep"() -> (w738:dbl)
                        n125 = Multiply(x=-1.0, y=w738) -> (x*y=w740:dbl)
                        n126 = call <userlib>:"LSX Move Rel.vi"("bWait"=w736, "dA"=w736, "dZ"=w736, "error in (no error)"=w748, "dY"=w740, "dX"=w736, "lLSID"=w739) -> ("error out"=w742:errorcluster)  [unwired: 3 in, 1 out]
                        n127 = call <userlib>:"LSX Get Pos.vi"("lLSID"=w739, "error in (no error)"=w742) -> ("pdA out"=w743:dbl, "pdX out"=w746:dbl, "pdY out"=w745:dbl, "pdZ out"=w744:dbl, "error out"=w747:errorcluster)  [unwired: 8 in, 1 out]
                        n128 = Build Array(w746, w745, w744, w743) -> (w737:dbl[])
                        n129 = local write "TANGOPosition"(w737) -> ()
                      }
                    }
                  }
                  frame "LEFT" {
                    n130 = case shown="\"PRESSED\"" w752 {
                      tunnel: w750 -> [w753 w770]
                      tunnel: [w753 w769] -> w749
                      tunnel: w751 -> [_ w758]
                      frame "RELEASED", Default {
                      }
                      frame "PRESSED" {
                        w756 = 0  # lATimeoutValue (0:wait infinite)
                        w760 = 0.0 ("dY")
                        n131 = local read "TANGOStep"() -> (w763:dbl)
                        n132 = Multiply(x=-1.0, y=w763) -> (x*y=w761:dbl)
                        n133 = call <userlib>:"LSX Move Rel.vi"("bWait"=w760, "dA"=w760, "dZ"=w760, "error in (no error)"=w770, "dY"=w760, "dX"=w761, "lLSID"=w758) -> ("error out"=w759:errorcluster)  [unwired: 3 in, 1 out]
                        n134 = call <userlib>:"LSX Wait For Axis Stop.vi"("pbATimeout"=10000, "error in (no error)"=w759, "lATimeoutValue"=w756, "lAFlags"=i8 15, "lLSID"=w758) -> ("error out"=w757:errorcluster)  [unwired: 4 in, 2 out]
                        n135 = call <userlib>:"LSX Get Pos.vi"("lLSID"=w758, "error in (no error)"=w757) -> ("pdA out"=w765:dbl, "pdX out"=w768:dbl, "pdY out"=w767:dbl, "pdZ out"=w766:dbl, "error out"=w769:errorcluster)  [unwired: 8 in, 1 out]
                        n136 = Build Array(w768, w767, w766, w765) -> (w762:dbl[])
                        n137 = local write "TANGOPosition"(w762) -> ()
                      }
                    }
                  }
                  frame "RIGHT" {
                    n138 = case shown="\"RELEASED\", Default" w774 {
                      tunnel: w772 -> [w775 w788]
                      tunnel: [w775 w787] -> w771
                      tunnel: w773 -> [_ w780]
                      frame "RELEASED", Default {
                      }
                      frame "PRESSED" {
                        w776 = 0.0 ("dY")
                        n139 = local read "TANGOStep"() -> (w779:dbl)
                        n140 = Multiply(x=1.0, y=w779) -> (x*y=w777:dbl)
                        n141 = call <userlib>:"LSX Move Rel.vi"("bWait"=w776, "dA"=w776, "dZ"=w776, "error in (no error)"=w788, "dY"=w776, "dX"=w777, "lLSID"=w780) -> ("error out"=w782:errorcluster)  [unwired: 3 in, 1 out]
                        n142 = call <userlib>:"LSX Get Pos.vi"("lLSID"=w780, "error in (no error)"=w782) -> ("pdA out"=w783:dbl, "pdX out"=w786:dbl, "pdY out"=w785:dbl, "pdZ out"=w784:dbl, "error out"=w787:errorcluster)  [unwired: 8 in, 1 out]
                        n143 = Build Array(w786, w785, w784, w783) -> (w778:dbl[])
                        n144 = local write "TANGOPosition"(w778) -> ()
                      }
                    }
                  }
                  frame "SAVEPOS" {
                    n145 = local read "IX 81 Port"() -> (w804:refnum<visa-resource-name>)
                    n146 = call <userlib>:"LSX Get Pos.vi"("lLSID"=w811, "error in (no error)"=w805) -> ("pdX out"=w810:dbl, "pdY out"=w809:dbl, "error out"=w802:errorcluster)  [unwired: 8 in, 3 out]
                    n147 = call "OlympusQuery.vi"("error in (no error)"=w805, "Device Number\n(1: -Condensor\n     - Objective\n     - Lamp\n     - Shutter\n2: - Z-Motion\n   - Autofocus)"=2 ("Device Number\n(1: -Condensor\n     - Objective\n     - Lamp\n     - Shutter\n2: - Z-Motion\n   - Autofocus)"), "String"="POS?", "VISA Resource Name In"=w804) -> ("error out"=w793:errorcluster, "Result"=w803:string)  [unwired: 5 in, 1 out]
                    n148 = Merge Errors(w802, w793) -> (w801:errorcluster)
                    n149 = Decimal String To Number(string=w803, default (0L)=0.0 ("default (0 I32)")) -> (number=w795:dbl)  [unwired: 1 in, 1 out]
                    n150 = Divide(x=w795, y=1000.0) -> (x/y=w796:dbl)
                    n151 = Bundle("pdX out"=w810, "pdY out"=w809, w796) -> (w800:cluster{"pdX out":dbl, "pdY out":dbl, dbl})  [unwired: 1 in]
                    n152 = Build Array(w800) -> (w792:cluster{"pdX out":dbl, "pdY out":dbl, dbl}[])
                    n153 = property on="PosList" class="MCListbox (strict)"() -> ("ItemNames"=w799:string[][])  [unwired: 2 in, 2 out]
                    n154 = call "TangoPositions2MultiList.vi"("error in (no error)"=w801, "Saved Positions"=w792) -> ("error out"=w790:errorcluster, "Array"=w798:string[][])  [unwired: 8 in]
                    n155 = Build Array (concatenate)(w799, w798) -> (w797:string[][])
                    n156 = property on="PosList" class="MCListbox (strict)"("ItemNames"=w797) -> ()  [unwired: 2 in, 2 out]
                    n157 = property on="PosListCapture" class="Bool (strict)"(error in=w790, "Value"=FALSE ("Save Pos")) -> (error out=w789:errorcluster)  [unwired: 1 in, 1 out]
                  }
                  frame "CLEARPOS" {
                    n158 = property on="PosList" class="MCListbox (strict)"(error in=w816) -> (error out=w815:errorcluster, "ItemNames"=w821:string[][])  [unwired: 1 in, 1 out]
                    n159 = Array Size(array=w821) -> (size(s)=w819:i32[])
                    n160 = Index Array(array=w819, index=0) -> (element=w818:i32)
                    n161 = Decrement(x=w818) -> (x-1=w822:i32)
                    n162 = Delete From Array(array=w821, index (row)=w822) -> (array with subset deleted=w817:string[][])  [unwired: 2 in, 1 out]
                    n163 = property on="PosList" class="MCListbox (strict)"(error in=w815, "ItemNames"=w817) -> (error out=w813:errorcluster)  [unwired: 1 in, 1 out]
                    n164 = property on="PosListClearLast" class="Bool (strict)"(error in=w813, "Value"=FALSE ("Clear Last Pos")) -> (error out=w812:errorcluster)  [unwired: 1 in, 1 out]
                  }
                  frame "SELECTPOS" {
                    n165 = property on="PosList" class="MCListbox (strict)"(error in=w825) -> (error out=w824:errorcluster, "ItemNames"=w828:string[][])  [unwired: 1 in, 1 out]
                    n166 = call "TangoSelectPos.vi"("TANGO ID"=w826, "error in (no error)"=w824, "Button"=w827, "ItemNames"=w828) -> ("error out"=w823:errorcluster)  [unwired: 7 in]
                  }
                  frame "EXPORT" {
                    n167 = property on="PosList" class="MCListbox (strict)"(error in=w832) -> (error out=w833:errorcluster, "ItemNames"=w834:string[][])  [unwired: 1 in, 1 out]
                    n168 = call "ConfigExportPosList.vi"("Array"=w834, "error in (no error)"=w833) -> ("error out"=w831:errorcluster)  [unwired: 7 in, 1 out]
                    n169 = property on="PosListSaveXML" class="Bool (strict)"(error in=w831, "Value"=FALSE ("Save Pos List")) -> (error out=w830:errorcluster)  [unwired: 1 in, 1 out]
                  }
                  frame "CALIBRATE" {
                    n170 = call "TangoCalibrate.vi"("error in (no error)"=w841, "plLSID in"=w840) -> ("error out"=w836:errorcluster, "X Limits"=w839:dbl[], "Y Limits"=w838:dbl[])  [unwired: 7 in]
                    n171 = local write "TANGOxLimits"(w838) -> ()
                    n172 = local write "TANGOyLimits"(w839) -> ()
                    n173 = property on="TANGOCalibrate" class="Bool (strict)"(error in=w836, "Value"=FALSE ("Tango Calibrate")) -> (error out=w835:errorcluster)  [unwired: 1 in, 1 out]
                  }
                }
              }
              n174 = while {
                tunnel: w197 -> [w847]
                tunnel: [w850] -> w158
                tunnel: 5 -> [w842]
                tunnel: w177 -> [w846]
                tunnel: [w848] -> w155
                stop <- w849 stop-if-true
                # "TANGO Stage Message Loop"
                n175 = event shown="[0] Timeout" {
                  selector: _ -> [_ _ _ _ _ _ _ _ _ _]
                  dyn-events: _ -> [_ _ _ _ _ _ _ _ _ _]
                  timeout: w842 -> [_ _ _ _ _ _ _ _ _ _]
                  tunnel: w846 -> [w852 w855 w861 w869 w885 w892 w897 w909 w921 w931]
                  tunnel: [w852 w856 w864 w870 w884 w891 w899 w911 w924 w933] -> w848
                  tunnel: [w851 w857 w863 w871 w883 w890 w900 w912 w925 w934] -> w850
                  tunnel: w847 -> [w851 w854 w862 w872 w881 w889 w898 w910 w922 w932]
                  event Timeout {
                    n176 = event-data() -> ()  [unwired: 1 in, 3 out]
                  }
                  event "TANGOUp": Value Change {
                    n177 = event-data() -> ("NewVal"=w853:bool)  [unwired: 1 in, 5 out]
                    n178 = case shown="False" w853 {
                      tunnel: ["UP RELEASED" "UP PRESSED"] -> w858
                      frame False {
                      }
                      frame True {
                      }
                    }
                    n179 = Enqueue Element(queue=w854, element=w858, error in (no error)=w855) -> (queue out=w857:refnum<queue>, error out=w856:errorcluster)  [unwired: 1 in, 1 out]
                  }
                  event "TANGODown": Value Change {
                    n180 = event-data() -> ("NewVal"=w865:bool)  [unwired: 1 in, 5 out]
                    n181 = case shown="True" w865 {
                      tunnel: ["DOWN RELEASED" "DOWN PRESSED"] -> w866
                      frame False {
                      }
                      frame True {
                      }
                    }
                    n182 = Enqueue Element(queue=w862, element=w866, error in (no error)=w861) -> (queue out=w863:refnum<queue>, error out=w864:errorcluster)  [unwired: 1 in, 1 out]
                  }
                  event "TANGOCalibrate": Value Change {
                    n183 = event-data() -> ("NewVal"=w873:bool)  [unwired: 1 in, 5 out]
                    n184 = case shown="True" w873 {
                      tunnel: w872 -> [w875 w877]
                      tunnel: [w875 w880] -> w871
                      tunnel: [w874 w879] -> w870
                      tunnel: w869 -> [w874 w878]
                      frame False {
                      }
                      frame True {
                        n185 = Enqueue Element(queue=w877, element="CALIBRATE", error in (no error)=w878) -> (queue out=w880:refnum<queue>, error out=w879:errorcluster)  [unwired: 1 in, 1 out]
                      }
                    }
                  }
                  event "TANGOLeft": Value Change {
                    n186 = event-data() -> ("NewVal"=w882:bool)  [unwired: 1 in, 5 out]
                    n187 = case shown="True" w882 {
                      tunnel: ["LEFT RELEASED" "LEFT PRESSED"] -> w886
                      frame False {
                      }
                      frame True {
                      }
                    }
                    n188 = Enqueue Element(queue=w881, element=w886, error in (no error)=w885) -> (queue out=w883:refnum<queue>, error out=w884:errorcluster)  [unwired: 1 in, 1 out]
                  }
                  event "TANGORight": Value Change {
                    n189 = event-data() -> ("NewVal"=w894:bool)  [unwired: 1 in, 5 out]
                    n190 = case shown="True" w894 {
                      tunnel: ["RIGHT RELEASED" "RIGHT PRESSED"] -> w893
                      frame False {
                      }
                      frame True {
                      }
                    }
                    n191 = Enqueue Element(queue=w889, element=w893, error in (no error)=w892) -> (queue out=w890:refnum<queue>, error out=w891:errorcluster)  [unwired: 1 in, 1 out]
                  }
                  event "PosListCapture": Value Change {
                    n192 = event-data() -> ("NewVal"=w901:bool)  [unwired: 1 in, 5 out]
                    n193 = case shown="True" w901 {
                      tunnel: [w905 w907] -> w900
                      tunnel: [w904 w908] -> w899
                      tunnel: w898 -> [w903 w907]
                      tunnel: w897 -> [w902 w908]
                      frame True {
                        n194 = Enqueue Element(queue=w903, element="SAVEPOS", error in (no error)=w902) -> (queue out=w905:refnum<queue>, error out=w904:errorcluster)  [unwired: 1 in, 1 out]
                      }
                      frame False {
                      }
                    }
                  }
                  event "PosListClearLast": Value Change {
                    n195 = event-data() -> ("NewVal"=w913:bool)  [unwired: 1 in, 5 out]
                    n196 = case shown="True" w913 {
                      tunnel: [w917 w919] -> w912
                      tunnel: [w916 w920] -> w911
                      tunnel: w910 -> [w915 w919]
                      tunnel: w909 -> [w914 w920]
                      frame True {
                        n197 = Enqueue Element(queue=w915, element="CLEARPOS", error in (no error)=w914) -> (queue out=w917:refnum<queue>, error out=w916:errorcluster)  [unwired: 1 in, 1 out]
                      }
                      frame False {
                      }
                    }
                  }
                  event "PosList": Value Change {
                    n198 = event-data() -> ("NewVal"=w929:i32[])  [unwired: 1 in, 5 out]
                    n199 = Number To Decimal String(number=w929) -> (decimal integer string=w927:string[])  [unwired: 1 in]
                    n200 = call <vilib>:"Space Constant.vi"() -> ("String"=w928:string)
                    n201 = Concatenate Strings("SELECTPOS", w928, w927) -> (w923:string)
                    n202 = Enqueue Element(queue=w922, element=w923, error in (no error)=w921) -> (queue out=w925:refnum<queue>, error out=w924:errorcluster)  [unwired: 1 in, 1 out]
                  }
                  event "PosListSaveXML": Value Change {
                    n203 = event-data() -> ("NewVal"=w930:bool)  [unwired: 1 in, 5 out]
                    n204 = case shown="False" w930 {
                      tunnel: [w936 w941] -> w934
                      tunnel: [w935 w940] -> w933
                      tunnel: w932 -> [w936 w939]
                      tunnel: w931 -> [w935 w938]
                      frame False {
                      }
                      frame True {
                        n205 = Enqueue Element(queue=w939, element="EXPORT XML", error in (no error)=w938) -> (queue out=w941:refnum<queue>, error out=w940:errorcluster)  [unwired: 1 in, 1 out]
                      }
                    }
                  }
                }
                n206 = local read "ProgramCreate"() -> (w844:bool)
                n207 = local read "ProgramRun"() -> (w843:bool)
                n208 = local read "ProgramStop"() -> (w845:bool)
                n209 = Compound Arithmetic op=OR(w848, w845, w844, w843) -> (w849:bool)
              }
              n210 = while {
                tunnel: w200 -> [w605]
                tunnel: [w606] -> w198
                tunnel: 5 -> [w601]
                tunnel: w199 -> [w604]
                tunnel: [w609] -> w139
                stop <- w608 stop-if-true
                # "Fluid Message Handling Loop"
                n211 = local read "ProgramCreate"() -> (w603:bool)
                n212 = event shown="[7] \"ValveFlushOn\": Value Change" {
                  selector: _ -> [_ _ _ _ _ _ _ _ _ _]
                  dyn-events: _ -> [_ _ _ _ _ _ _ _ _ _]
                  timeout: w601 -> [_ _ _ _ _ _ _ _ _ _]
                  tunnel: w604 -> [w611 w612 w625 w640 w657 w662 w667 w670 w690 w698]
                  tunnel: [w611 w614 w628 w643 w655 w660 w665 w673 w691 w701] -> w609
                  tunnel: [w610 w615 w627 w642 w656 w661 w666 w672 w692 w702] -> w606
                  tunnel: w605 -> [w610 w613 w626 w641 w658 w663 w668 w671 w689 w700]
                  event Timeout {
                    n213 = event-data() -> ()  [unwired: 1 in, 3 out]
                  }
                  event "CalibStart": Value Change {
                    n214 = event-data() -> ("NewVal"=w616:bool)  [unwired: 1 in, 5 out]
                    n215 = case shown="True" w616 {
                      tunnel: [w618 w623] -> w615
                      tunnel: [w617 w622] -> w614
                      tunnel: w613 -> [w618 w620]
                      tunnel: w612 -> [w617 w619]
                      frame False {
                      }
                      frame True {
                        n216 = Enqueue Element(queue=w620, element="CALIBRATE", error in (no error)=w619) -> (queue out=w623:refnum<queue>, error out=w622:errorcluster)  [unwired: 1 in, 1 out]
                      }
                    }
                  }
                  event "ValveFeedOn": Value Change {
                    n217 = event-data() -> ("NewVal"=w624:bool)  [unwired: 1 in, 5 out]
                    n218 = case shown="True" w624 {
                      tunnel: [w629 w634] -> w628
                      tunnel: [w630 w635] -> w627
                      tunnel: w626 -> [w630 w638]
                      tunnel: w625 -> [w629 w637]
                      frame False {
                      }
                      frame True {
                        n219 = Enqueue Element(queue=w638, element="FEED", error in (no error)=w637) -> (queue out=w632:refnum<queue>, error out=w633:errorcluster)  [unwired: 1 in, 1 out]
                        n220 = Enqueue Element(queue=w632, element="CLOSE ALL", error in (no error)=w633) -> (queue out=w635:refnum<queue>, error out=w634:errorcluster)  [unwired: 1 in, 1 out]
                      }
                    }
                  }
                  event "ValvePumpOn": Value Change {
                    n221 = event-data() -> ("NewVal"=w639:bool)  [unwired: 1 in, 5 out]
                    n222 = case shown="True" w639 {
                      tunnel: [w644 w649] -> w643
                      tunnel: [w645 w650] -> w642
                      tunnel: w641 -> [w645 w653]
                      tunnel: w640 -> [w644 w652]
                      frame False {
                      }
                      frame True {
                        n223 = Enqueue Element(queue=w653, element="PUMP", error in (no error)=w652) -> (queue out=w647:refnum<queue>, error out=w648:errorcluster)  [unwired: 1 in, 1 out]
                        n224 = Enqueue Element(queue=w647, element="CLOSE ALL", error in (no error)=w648) -> (queue out=w650:refnum<queue>, error out=w649:errorcluster)  [unwired: 1 in, 1 out]
                      }
                    }
                  }
                  event "A1", "A2", "A3", "A4", "A5", "A6", "A7", "A8", "B1", "B3", "B4", "B5", "B2", "B6", "B7", "B8", "C1", "C2", "C3", "C4", "C5", "C6", "C7", "C8": Value Change {
                    n225 = event-data() -> ()  [unwired: 1 in, 6 out]
                    n226 = Enqueue Element(queue=w658, element="SINGLE VALVE", error in (no error)=w657) -> (queue out=w656:refnum<queue>, error out=w655:errorcluster)  [unwired: 1 in, 1 out]
                  }
                  event "ValveCloseAll": Value Change {
                    n227 = event-data() -> ()  [unwired: 1 in, 6 out]
                    n228 = Enqueue Element(queue=w663, element="CLOSE ALL", error in (no error)=w662) -> (queue out=w661:refnum<queue>, error out=w660:errorcluster)  [unwired: 1 in, 1 out]
                  }
                  event "ValveOpenAll": Value Change {
                    n229 = event-data() -> ()  [unwired: 1 in, 6 out]
                    n230 = Enqueue Element(queue=w668, element="OPEN ALL", error in (no error)=w667) -> (queue out=w666:refnum<queue>, error out=w665:errorcluster)  [unwired: 1 in, 1 out]
                  }
                  event "ValveFlushOn": Value Change {
                    n231 = event-data() -> ("NewVal"=w669:bool)  [unwired: 1 in, 5 out]
                    n232 = case shown="False" w669 {
                      tunnel: [w678 w680] -> w673
                      tunnel: [w677 w679] -> w672
                      tunnel: w671 -> [w676 w686]
                      tunnel: w670 -> [w675 w685]
                      frame True {
                        n233 = Enqueue Element(queue=w676, element="FLUSH ON", error in (no error)=w675) -> (queue out=w677:refnum<queue>, error out=w678:errorcluster)  [unwired: 1 in, 1 out]
                      }
                      frame False, Default {
                        n234 = Enqueue Element(queue=w686, element="FLUSH OFF", error in (no error)=w685) -> (queue out=w682:refnum<queue>, error out=w681:errorcluster)  [unwired: 1 in, 1 out]
                        n235 = Enqueue Element(queue=w682, element="CLOSE ALL", error in (no error)=w681) -> (queue out=w679:refnum<queue>, error out=w680:errorcluster)  [unwired: 1 in, 1 out]
                      }
                    }
                  }
                  event "ProgramSingleMultiring": Value Change {
                    n236 = event-data() -> ("NewVal"=w688:bool)  [unwired: 1 in, 5 out]
                    n237 = case shown="False" w688 {
                      tunnel: ["MULTIRING" ("element") "ONERING" ("element")] -> w687
                      frame True {
                      }
                      frame False {
                      }
                    }
                    n238 = Enqueue Element(queue=w689, element=w687, error in (no error)=w690) -> (queue out=w692:refnum<queue>, error out=w691:errorcluster)  [unwired: 1 in, 1 out]
                  }
                  event "CalibRestart": Value Change {
                    n239 = event-data() -> ()  [unwired: 1 in, 6 out]
                    n240 = property on="CalibRestart" class="Bool (strict)"("Value"=FALSE ("CalibRestart")) -> ()  [unwired: 2 in, 2 out]
                    n241 = property on="CalibStart" class="Bool (strict)"(error in=w698, "BoolText.Text"="Restart Calibration" ("Boolean Text.Text")) -> (error out=w697:errorcluster)  [unwired: 1 in, 1 out]
                    n242 = Enqueue Element(queue=w700, element="CALIBRATE", error in (no error)=w697) -> (queue out=w702:refnum<queue>, error out=w701:errorcluster)  [unwired: 1 in, 1 out]
                  }
                }
                n243 = local read "ProgramRun"() -> (w602:bool)
                n244 = local read "ProgramStop"() -> (w607:bool)
                n245 = Compound Arithmetic op=OR(w609, w607, w603, w602) -> (w608:bool)
              }
              n246 = while {
                tunnel: w205 -> [w345]
                tunnel: 1000 -> [w340]
                tunnel: w177 -> [w339]
                tunnel: [w338] -> w176
                stop <- w344 stop-if-true
                # "Position Measurement"
                n247 = event shown="[0] Timeout" {
                  selector: _ -> [_]
                  dyn-events: _ -> [_]
                  timeout: w340 -> [_]
                  tunnel: w345 -> [w348]
                  tunnel: [w347] -> w338
                  tunnel: w339 -> [w346]
                  event Timeout {
                    n248 = event-data() -> ()  [unwired: 1 in, 3 out]
                    n249 = call <userlib>:"LSX Get Pos.vi"("lLSID"=w348, "error in (no error)"=w346) -> ("pdA out"=w350:dbl, "pdX out"=w353:dbl, "pdY out"=w352:dbl, "pdZ out"=w351:dbl, "error out"=w347:errorcluster)  [unwired: 8 in, 1 out]
                    n250 = Build Array(w353, w352, w351, w350) -> (w349:dbl[])
                    n251 = local write "TANGOPosition"(w349) -> ()
                  }
                }
                n252 = local read "ProgramCreate"() -> (w341:bool)
                n253 = local read "ProgramRun"() -> (w342:bool)
                n254 = local read "ProgramStop"() -> (w343:bool)
                n255 = Compound Arithmetic op=OR(w338, w343, w342, w341) -> (w344:bool)
              }
              n256 = while {
                tunnel: w185 -> [w213]
                shift-right: [w208] -> w161
                shift-left: w163 -> [w209]
                tunnel: w146 -> [w212]
                tunnel: [w207] -> w144
                stop <- w207 stop-if-true
                # "ANDOR Camera Execution Loop"
                n257 = Dequeue Element(queue=w213, error in (no error)=w212) -> (element=w211:string, error out=w210:errorcluster)  [unwired: 1 in, 2 out]
                n258 = Wait (ms)(milliseconds to wait=u32 50) -> ()  [unwired: 1 out]
                n259 = case shown="\"AUTOHISTOGRAM\"" w211 {
                  tunnel: w210 -> [w216 w227 w233 w243 w252 w256 w266]
                  tunnel: [w215 w226 w232 w242 w253 w256 w265] -> w207
                  tunnel: w209 -> [w214 w223 w231 w240 w249 w255 w260]
                  tunnel: [w214 w223 w230 w240 w249 w255 w264] -> w208
                  frame "SAVESINGLEIMAGE" {
                    n260 = local read "ANDORImgName"() -> (w221:string)
                    n261 = local read "ANDORColormap"() -> (w220:u16)
                    n262 = local read "ANDORImgFormat"() -> (w219:u16)
                    n263 = local read "ANDORImgPath"() -> (w218:path)
                    n264 = call "AndorAcqSingleImgToFile.vi"("Image Name"=w221, "Image Path"=w218, "error in (no error)"=w216, "Colormap"=w220, "Format"=w219) -> ("error out"=w222:errorcluster)  [unwired: 6 in]
                    n265 = property on="ANDORImgSave" class="Bool (strict)"(error in=w222, "Value"=FALSE ("Save Image")) -> (error out=w215:errorcluster)  [unwired: 1 in, 1 out]
                  }
                  frame "EXPOSURE" {
                    n266 = call "AndorIdle.vi"("error in (no error)"=w227) -> ("error out"=w224:errorcluster)  [unwired: 9 in, 1 out]
                    n267 = local read "ANDORExposure"() -> (w225:sgl)
                    n268 = Divide(x=w225, y=sgl 1000.0) -> (x/y=w229:sgl)
                    n269 = call "Set Exposure Time.vi"("error in (no error)"=w224, "time"=w229) -> ("error out"=w226:errorcluster)  [unwired: 8 in, 1 out]
                  }
                  frame "SINGLEIMAGE" {
                    n270 = local read "ANDORExposure"() -> (w235:sgl)
                    n271 = property on="ANDORImage" class="ImageControl"() -> ("Image Area Height"=w236:u32, "Image Area Width"=w237:u32)  [unwired: 2 in, 2 out]
                    n272 = call "AndorAcqSingleImgToIMAQ.vi"("IMAQ In"=w231, "error in (no error)"=w233, "Exposure Time"=w235, "Image Area Width"=w237, "Image Area Height"=w236) -> ("error out"=w238:errorcluster, "Image Dst Out"=w230:T8)  [unwired: 5 in]
                    n273 = property on="ANDORImgSingle" class="Bool (strict)"(error in=w238, "Value"=FALSE ("Single Image")) -> (error out=w232:errorcluster)  [unwired: 1 in, 1 out]
                    n274 = local write "ANDORImage"(w230) -> ()
                  }
                  frame "HISTOGRAM" {
                    w245 = T12 7 items=["Grayscale (U8)", "Grayscale (I16)", "Grayscale (SGL)", "Complex (CSG)", "RGB (U32)", "HSL (U32)", "RGB (U64)", "Grayscale (U16)"] ("Image Type")
                    n275 = call "IMAQ Create"("Image Name"="AdjustedImage", "Image Type"=w245, "error in (no error)"=w243) -> ("New Image"=w239:T8, "error out"=w241:errorcluster)  [unwired: 2 in]
                    n276 = local read "AndorHistRange"() -> (w247:cluster{"Minimum":sgl, "Maximum":sgl})
                    n277 = call "IMAQ MathLookup"("Range"=w247, "Operator"=T10."Linear", "error in (no error)"=w241, "Image Dst"=w239, "Image Src"=w240) -> ("error out"=w242:errorcluster, "Image Dst Out"=w248:T8)  [unwired: 5 in]
                    n278 = local write "ANDORImage"(w248) -> ()
                  }
                  frame "AUTOHISTOGRAM" {
                    n279 = call "IMAQ Histogram"("error in (no error)"=w252, "Image"=w249) -> ("error out"=w253:errorcluster, "Histogram Report"=w254:T13)  [unwired: 8 in]
                    n280 = Unbundle By Name(w254) -> ("Minimal Value"=w250:sgl, "Maximal Value"=w251:sgl)
                    n281 = property on="Minimum" class="Slide (strict)"("Minimum"=w250, "Maximum"=w251, "Scale.Maximum"=w251, "Scale.Minimum"=w250, "Value"=w250) -> ()  [unwired: 2 in, 2 out]
                    n282 = property on="Maximum" class="Slide (strict)"("Maximum"=w251, "Minimum"=w250, "Scale.Maximum"=w251, "Scale.Minimum"=w250, "Value"=w251) -> ()  [unwired: 2 in, 2 out]
                  }
                  frame "", Default {
                  }
                  frame "LIVE" {
                    w270 = 5  # Run till abort
                    w268 = 4  # Image
                    n283 = property on="ANDORExposure" class="DigNum (strict)"(error in=w266, "DisabledEnum"=T9."Disabled and Grayed Out" ("Disabled")) -> (error out=w273:errorcluster)  [unwired: 1 in, 1 out]
                    n284 = call "Set Read Mode.vi"("error in (no error)"=w273, "mode"=w268) -> ("error out"=w274:errorcluster)  [unwired: 8 in, 1 out]
                    n285 = call "Set Kinetic Cycle Time.vi"("error in (no error)"=w274, "time"=sgl 0.0) -> ("error out"=w275:errorcluster)  [unwired: 8 in, 1 out]
                    n286 = call "Set Acquisition Mode.vi"("error in (no error)"=w275, "mode"=w270) -> ("error out"=w262:errorcluster)  [unwired: 8 in, 1 out]
                    n287 = call "AndorIdle.vi"("error in (no error)"=w262) -> ("error out"=w263:errorcluster)  [unwired: 9 in, 1 out]
                    n288 = control-ref of="ANDORImage"() -> (w258:refnum<vi>)
                    n289 = call "Start Acquisition.vi"("error in (no error)"=w263) -> ("error out"=w261:errorcluster)  [unwired: 9 in, 1 out]
                    n290 = property on="Property Node" class="ImageControl"(reference=w258) -> ("Image Area Size"=w259:cluster{"Width":u32, "Height":u32})  [unwired: 1 in, 2 out]
                    n291 = control-ref of="AndorHistRange"() -> (w257:refnum<vi>)
                    n292 = while {
                      tunnel: [w286] -> w264
                      tunnel: w260 -> [w287]
                      tunnel: w261 -> [w288]
                      tunnel: [w281] -> w276
                      tunnel: w259 -> [w280]
                      tunnel: w257 -> [w279]
                      stop <- w285 stop-if-true
                      # "Live Mode Loop"
                      n293 = local read "ANDORLive"() -> (w283:bool)
                      n294 = local read "ProgramStop"() -> (w282:bool)
                      n295 = call "AndorLiveMode.vi"("error in (no error)"=w288, "Image Area:Size:All Elements"=w280, "AndorHistRange"=w279, "Imaq In"=w287) -> ("error out"=w281:errorcluster, "Image"=w286:T8)  [unwired: 6 in]
                      n296 = Not(x=w283) -> (.not. x?=w284:bool)
                      n297 = local write "ANDORImage"(w286) -> ()
                      n298 = Compound Arithmetic op=OR(w281, w282, w284) -> (w285:bool)
                    }
                    n299 = call "Abort Acquisition.vi"("error in (no error)"=w276) -> ("error out"=w277:errorcluster)  [unwired: 9 in, 1 out]
                    n300 = property on="ANDORLive" class="Bool (strict)"(error in=w277, "Value"=FALSE ("Live Mode")) -> (error out=w278:errorcluster)  [unwired: 1 in, 1 out]
                    n301 = property on="ANDORExposure" class="DigNum (strict)"(error in=w278, "DisabledEnum"=T9."Enabled" ("Disabled")) -> (error out=w265:errorcluster)  [unwired: 1 in, 1 out]
                  }
                }
              }
              n302 = while {
                tunnel: w196 -> [w1168]
                tunnel: [w1171] -> w204
                tunnel: 100 -> [w1161]
                tunnel: 5 -> [w1160]
                tunnel: w148 -> [w1167]
                tunnel: [w1165] -> w153
                stop <- w1170 stop-if-true
                # "Microscope Control Queue"
                n303 = event shown="[0] Timeout" {
                  selector: _ -> [_]
                  dyn-events: _ -> [_]
                  timeout: w1161 -> [_]
                  tunnel: w1168 -> [w1175]
                  tunnel: w1167 -> [w1174]
                  tunnel: [w1173] -> w1164
                  event Timeout {
                    n304 = event-data() -> ()  [unwired: 1 in, 3 out]
                    n305 = Enqueue Element(queue=w1175, element=cluster{"Button":string, "Value":dbl} {"Button"="FOCUSUPDATE", "Value"=0.0}, error in (no error)=w1174) -> (error out=w1173:errorcluster)  [unwired: 1 in, 2 out]
                  }
                }
                n306 = event shown="[8] \"IX81Filter\": Value Change" {
                  selector: _ -> [_ _ _ _ _ _ _ _ _]
                  dyn-events: _ -> [_ _ _ _ _ _ _ _ _]
                  timeout: w1160 -> [_ _ _ _ _ _ _ _ _]
                  tunnel: w1167 -> [w1180 w1185 w1195 w1200 w1208 w1216 w1224 w1233 w1238]
                  tunnel: [w1179 w1183 w1193 w1198 w1206 w1214 w1222 w1231 w1236] -> w1166
                  tunnel: w1168 -> [w1181 w1186 w1196 w1201 w1209 w1217 w1225 w1234 w1239]
                  tunnel: [w1178 w1184 w1194 w1199 w1207 w1215 w1223 w1232 w1237] -> w1171
                  event Timeout {
                    n307 = event-data() -> ()  [unwired: 1 in, 3 out]
                    n308 = Get Queue Status(queue=w1181, return elements? (F)=TRUE, error in (no error)=w1180) -> (queue out=w1178:refnum<queue>, error out=w1179:errorcluster, elements=→"elements":cluster{"Button":string, "Value":dbl}[])  [unwired: 5 out]
                  }
                  event "IX81Intensity": Value Change {
                    n309 = event-data() -> ("NewVal"=w1187:dbl)  [unwired: 1 in, 5 out]
                    n310 = Bundle("INTENSITY", "NewVal"=w1187) -> (w1182:cluster{string, "NewVal":dbl})  [unwired: 1 in]
                    n311 = Enqueue Element(queue=w1186, element=w1182, error in (no error)=w1185) -> (queue out=w1184:refnum<queue>, error out=w1183:errorcluster)  [unwired: 1 in, 1 out]
                  }
                  event "IX81Prism": Value Change {
                    n312 = event-data() -> ("NewVal"=w1191:u16)  [unwired: 1 in, 5 out]
                    n313 = To Double Precision Float(number=w1191) -> (double precision float=w1189:dbl)
                    n314 = Bundle("PRISM", w1189) -> (w1190:cluster{string, dbl})  [unwired: 1 in]
                    n315 = Enqueue Element(queue=w1196, element=w1190, error in (no error)=w1195) -> (queue out=w1194:refnum<queue>, error out=w1193:errorcluster)  [unwired: 1 in, 1 out]
                  }
                  event "IX81Objective": Value Change {
                    n316 = event-data() -> ("NewVal"=w1203:enum16{"x 4", "x 10", "x 20", "x 40", "x 100"})  [unwired: 1 in, 5 out]
                    n317 = Bundle("OBJECTIVE", "NewVal"=w1203) -> (w1197:T14)  [unwired: 1 in]
                    n318 = Enqueue Element(queue=w1201, element=w1197, error in (no error)=w1200) -> (queue out=w1199:refnum<queue>, error out=w1198:errorcluster)  [unwired: 1 in, 1 out]
                  }
                  event "IX81SettingsAppend": Value Change {
                    n319 = event-data() -> ("NewVal"=w1211:bool)  [unwired: 1 in, 5 out]
                    n320 = Boolean To (0,1)(Boolean=w1211) -> (0, 1=w1204:i16)
                    n321 = Bundle("APPEND SETTINGS", w1204) -> (w1205:cluster{string, i16})  [unwired: 1 in]
                    n322 = Enqueue Element(queue=w1209, element=w1205, error in (no error)=w1208) -> (queue out=w1207:refnum<queue>, error out=w1206:errorcluster)  [unwired: 1 in, 1 out]
                  }
                  event "IX81SettingsSave": Value Change {
                    n323 = event-data() -> ("NewVal"=w1219:bool)  [unwired: 1 in, 5 out]
                    n324 = Boolean To (0,1)(Boolean=w1219) -> (0, 1=w1212:i16)
                    n325 = Bundle("SAVE SETTINGS", w1212) -> (w1213:cluster{string, i16})  [unwired: 1 in]
                    n326 = Enqueue Element(queue=w1217, element=w1213, error in (no error)=w1216) -> (queue out=w1215:refnum<queue>, error out=w1214:errorcluster)  [unwired: 1 in, 1 out]
                  }
                  event "IX81SettingsClear": Value Change {
                    n327 = event-data() -> ("NewVal"=w1227:bool)  [unwired: 1 in, 5 out]
                    n328 = Boolean To (0,1)(Boolean=w1227) -> (0, 1=w1220:i16)
                    n329 = Bundle("CLEAR SETTINGS", w1220) -> (w1221:cluster{string, i16})  [unwired: 1 in]
                    n330 = Enqueue Element(queue=w1225, element=w1221, error in (no error)=w1224) -> (queue out=w1223:refnum<queue>, error out=w1222:errorcluster)  [unwired: 1 in, 1 out]
                  }
                  event "IX81Focus": Value Change {
                    n331 = event-data() -> ("NewVal"=w1229:dbl)  [unwired: 1 in, 5 out]
                    n332 = Bundle("FOCUS", "NewVal"=w1229) -> (w1228:cluster{string, "NewVal":dbl})  [unwired: 1 in]
                    n333 = Enqueue Element(queue=w1234, element=w1228, error in (no error)=w1233) -> (queue out=w1232:refnum<queue>, error out=w1231:errorcluster)  [unwired: 1 in, 1 out]
                  }
                  event "IX81Filter": Value Change {
                    n334 = event-data() -> ("NewVal"=w1240:u16)  [unwired: 1 in, 5 out]
                    n335 = Bundle("FILTER", "NewVal"=w1240) -> (w1235:cluster{string, "NewVal":u16})  [unwired: 1 in]
                    n336 = Enqueue Element(queue=w1239, element=w1235, error in (no error)=w1238) -> (queue out=w1237:refnum<queue>, error out=w1236:errorcluster)  [unwired: 1 in, 1 out]
                  }
                }
                n337 = local read "ProgramCreate"() -> (w1163:bool)
                n338 = local read "ProgramRun"() -> (w1162:bool)
                n339 = local read "ProgramStop"() -> (w1169:bool)
                n340 = Merge Errors(w1164, w1166) -> (w1165:errorcluster)
                n341 = Compound Arithmetic op=OR(w1165, w1169, w1163, w1162) -> (w1170:bool)
              }
              n342 = while {
                tunnel: w200 -> [w361]
                tunnel: w201 -> [w357]
                tunnel: w199 -> [w360]
                tunnel: [w355] -> w130
                stop <- w355 stop-if-true
                # "Fluid Execution Loop"
                n343 = Dequeue Element(queue=w361, error in (no error)=w360) -> (queue out=w356:refnum<queue>, element=w359:string, error out=w358:errorcluster)  [unwired: 1 in, 1 out]
                n344 = Wait (ms)(milliseconds to wait=u32 50) -> ()  [unwired: 1 out]
                n345 = case shown="\"CALIBRATE\"" w359 {
                  tunnel: w358 -> [w369 w380 w386 w392 w395 w429 w446 w477 w593 w597]
                  tunnel: [w366 w375 w382 w388 w396 w426 w447 w475 w593 w597] -> w355
                  tunnel: w357 -> [w363 w377 w385 w391 w397 w430 w448 w471 _ _]
                  tunnel: w356 -> [_ _ _ _ _ w428 w445 _ _ _]
                  frame "FEED" {
                    n346 = local read "ProgramSingleMultiring"() -> (w372:bool)
                    n347 = local read "ValveFeedReagent"() -> (w368:u16)
                    n348 = local read "ValveFeedCycles"() -> (w370:i32)
                    n349 = local read "ValveFeedRingAll"() -> (w367:bool)
                    n350 = local read "ValveFeedRing"() -> (w371:u16)
                    n351 = call "ArdnoFeed.vi"("LINX Resource"=w363, "Single / Multiring?"=w372, "Channel"=w368, "Ring"=w371, "Feed Cycles"=w370, "error in (no error)"=w369, "All Rings"=w367, "Frequency"=u32 8) -> ("error out"=w365:errorcluster)  [unwired: 5 in, 2 out]
                    n352 = property on="ValveFeedOn" class="Bool (strict)"(error in=w365, "Value"=FALSE ("Feed On")) -> (error out=w366:errorcluster)  [unwired: 1 in, 1 out]
                  }
                  frame "PUMP" {
                    n353 = local read "ProgramSingleMultiring"() -> (w376:bool)
                    n354 = local read "ValvePumpFrequency"() -> (w379:dbl)
                    n355 = local read "ValvePumpCycles"() -> (w378:dbl)
                    n356 = call "ArdnoPump.vi"("LINX Resource"=w377, "Pump Cycles"=w378, "Pump Frequency"=w379, "error in (no error)"=w380, "Single/\nMultiring?"=w376) -> ("error out"=w374:errorcluster)  [unwired: 2 out]
                    n357 = property on="ValvePumpOn" class="Bool (strict)"(error in=w374, "Value"=FALSE ("Pump On")) -> (error out=w375:errorcluster)  [unwired: 1 in, 1 out]
                  }
                  frame "FLUSH ON", Default {
                    n358 = local read "ProgramSingleMultiring"() -> (w383:bool)
                    n359 = local read "ValveFlushReagent"() -> (w384:u16)
                    n360 = call "ArdnoFlush.vi"("Open?"=TRUE, "error in (no error)"=w386, "Single / Multivalve?"=w383, "Channel"=w384, "LINX Resource"=w385) -> ("error out"=w382:errorcluster)  [unwired: 5 in, 1 out]
                  }
                  frame "FLUSH OFF" {
                    n361 = local read "ProgramSingleMultiring"() -> (w389:bool)
                    n362 = local read "ValveFlushReagent"() -> (w390:u16)
                    n363 = call "ArdnoFlush.vi"("Open?"=FALSE, "error in (no error)"=w392, "Single / Multivalve?"=w389, "Channel"=w390, "LINX Resource"=w391) -> ("error out"=w388:errorcluster)  [unwired: 5 in, 1 out]
                  }
                  frame "SINGLE VALVE" {
                    n364 = Build Array("A1", "A2", "A3", "A4", "A5", "A6", "A7", "A8") -> (w401:bool[])
                    n365 = Build Array("B1", "B2", "B3", "B4", "B5", "B6", "B7", "B8") -> (w400:bool[])
                    n366 = Not(x=w401) -> (.not. x?=w394:bool[])
                    n367 = Build Array("C1", "C2", "C3", "C4", "C5", "C6", "C7", "C8") -> (w399:bool[])
                    n368 = Not(x=w399) -> (.not. x?=w393:bool[])
                    n369 = Build Array (concatenate)(w394, w400, w393) -> (w398:bool[])
                    n370 = call "ArdnoSingleValveControl.vi"("error in (no error)"=w395, "Array"=w398, "LINX Resource"=w397) -> ("Error Out"=w396:errorcluster)  [unwired: 7 in, 1 out]
                  }
                  frame "CLOSE ALL" {
                    n371 = case shown="True" "ValveCloseAll" {
                      tunnel: w430 -> [_ w442]
                      tunnel: [w433 w437] -> w426
                      tunnel: w429 -> [w434 w441]
                      tunnel: w428 -> [w431 _]
                      frame False {
                        n372 = Enqueue Element(queue=w431, element="SINGLE VALVE", error in (no error)=w434) -> (error out=w433:errorcluster)  [unwired: 1 in, 2 out]
                      }
                      frame True {
                        w435 = FALSE
                        w440 = FALSE
                        n373 = local read "ProgramSingleMultiring"() -> (w436:bool)
                        n374 = local write "C8"(w435) -> ()
                        n375 = local write "C7"(w435) -> ()
                        n376 = local write "C6"(w435) -> ()
                        n377 = local write "C5"(w435) -> ()
                        n378 = local write "C4"(w435) -> ()
                        n379 = local write "C3"(w435) -> ()
                        n380 = local write "C2"(w435) -> ()
                        n381 = local write "C1"(w435) -> ()
                        n382 = call "ArdnoAllValvesClosed.vi"("Single/Multiring?"=w436, "error in (no error)"=w441, "LINX Resource"=w442) -> ("error out"=w438:errorcluster)  [unwired: 7 in, 1 out]
                        n383 = local write "A3"(w440) -> ()
                        n384 = local write "A2"(w440) -> ()
                        n385 = local write "A1"(w440) -> ()
                        n386 = case shown="True" w436 {
                          frame False {
                          }
                          frame True {
                            w443 = FALSE
                            n387 = local write "A8"(w443) -> ()
                            n388 = local write "A7"(w443) -> ()
                            n389 = local write "A6"(w443) -> ()
                            n390 = local write "A5"(w443) -> ()
                            n391 = local write "A4"(w443) -> ()
                            n392 = local write "B8"(w443) -> ()
                            n393 = local write "B7"(w443) -> ()
                            n394 = local write "B6"(w443) -> ()
                            n395 = local write "B5"(w443) -> ()
                            n396 = local write "B4"(w443) -> ()
                            n397 = local write "B3"(w443) -> ()
                            n398 = local write "B2"(w443) -> ()
                            n399 = local write "B1"(w443) -> ()
                          }
                        }
                        n400 = property on="ValveCloseAll" class="Bool (strict)"(error in=w438, "Value"=FALSE ("Open all")) -> (error out=w437:errorcluster)  [unwired: 1 in, 1 out]
                      }
                    }
                  }
                  frame "OPEN ALL" {
                    n401 = case shown="True" "ValveOpenAll" {
                      tunnel: w448 -> [_ w460]
                      tunnel: [w451 w455] -> w447
                      tunnel: w446 -> [w452 w459]
                      tunnel: w445 -> [w449 _]
                      frame False {
                        n402 = Enqueue Element(queue=w449, element="SINGLE VALVE", error in (no error)=w452) -> (error out=w451:errorcluster)  [unwired: 1 in, 2 out]
                      }
                      frame True {
                        w458 = TRUE
                        w457 = TRUE
                        n403 = local read "ProgramSingleMultiring"() -> (w453:bool)
                        n404 = local write "C8"(w458) -> ()
                        n405 = local write "C7"(w458) -> ()
                        n406 = local write "C6"(w458) -> ()
                        n407 = local write "C5"(w458) -> ()
                        n408 = local write "C4"(w458) -> ()
                        n409 = local write "C3"(w458) -> ()
                        n410 = local write "C2"(w458) -> ()
                        n411 = local write "C1"(w458) -> ()
                        n412 = call "ArdnoAllValvesOpened.vi"("Single/\nMultiring?"=w453, "error in (no error)"=w459, "LINX Resource"=w460) -> ("error out"=w454:errorcluster)  [unwired: 7 in, 1 out]
                        n413 = local write "A3"(w457) -> ()
                        n414 = local write "A2"(w457) -> ()
                        n415 = local write "A1"(w457) -> ()
                        n416 = property on="ValveOpenAll" class="Bool (strict)"(error in=w454, "Value"=FALSE ("Open all")) -> (error out=w455:errorcluster)  [unwired: 1 in, 1 out]
                        n417 = case shown="True" w453 {
                          frame False {
                          }
                          frame True {
                            w461 = TRUE
                            n418 = local write "B8"(w461) -> ()
                            n419 = local write "B7"(w461) -> ()
                            n420 = local write "B6"(w461) -> ()
                            n421 = local write "B5"(w461) -> ()
                            n422 = local write "B4"(w461) -> ()
                            n423 = local write "B3"(w461) -> ()
                            n424 = local write "B2"(w461) -> ()
                            n425 = local write "B1"(w461) -> ()
                            n426 = local write "A8"(w461) -> ()
                            n427 = local write "A7"(w461) -> ()
                            n428 = local write "A6"(w461) -> ()
                            n429 = local write "A5"(w461) -> ()
                            n430 = local write "A4"(w461) -> ()
                          }
                        }
                      }
                    }
                  }
                  frame "CALIBRATE" {
                    n431 = property on="CalibStart" class="Bool (strict)"(error in=w477, "DisabledEnum"=T9."Disabled and Grayed Out" ("Disabled")) -> (error out=w472:errorcluster)  [unwired: 1 in, 1 out]
                    n432 = property on="CalibStart" class="Bool (strict)"(error in=w472) -> (error out=w468:errorcluster, "BoolText.Text"=w470:string)  [unwired: 1 in, 1 out]
                    n433 = local read "ProgramSingleMultiring"() -> (w463:bool)
                    n434 = local read "ANDORExposure"() -> (w469:sgl)
                    n435 = control-ref of="PosList"() -> (w464:refnum<vi>)
                    n436 = local read "TANGO"() -> (w465:i32)
                    n437 = case shown="\"Capture Full Intensity\"" w470 {
                      tunnel: w471 -> [_ _ w552 _]
                      tunnel: w469 -> [w485 w526 w553 _]
                      tunnel: [inf ("Number of pump steps\n for the desired refresh ratio") _ w550 _] -> w466
                      tunnel: [w484 w527 w549 w589] -> w467
                      tunnel: w468 -> [w483 w517 w535 w590]
                      tunnel: w463 -> [_ _ w547 _]
                      tunnel: w465 -> [w480 w524 w546 _]
                      tunnel: w464 -> [w479 w525 w545 _]
                      tunnel: T11."replace or create with confirmation" ("operation (0:open)") -> [w478 w512 w532 _]
                      frame "Capture Blank", Default {
                        n438 = call "Display Message to User"("error in (no error)"=w483) -> ("error out"=w482:errorcluster, "Sure"=w481:bool)  [unwired: 9 in]
                        n439 = case shown="True" w481 {
                          tunnel: w485 -> [_ w509]
                          tunnel: [w487 w505] -> w484
                          tunnel: w482 -> [w487 w492]
                          tunnel: w480 -> [_ w503]
                          tunnel: w479 -> [_ w502]
                          tunnel: w478 -> [_ w494]
                          frame False {
                          }
                          frame True {
                            n440 = Create Folder(prompt (Create Folder)="Specify the folder or type a new name to save the images in." ("prompt"), error in=w492) -> (created path=w490:path, error out=w493:errorcluster)  [unwired: 1 in, 1 out]
                            n441 = call <vilib>:"Clear Errors.vi"("error in (no error)"=w493, "specific error code to clear (0: all)"=10) -> ("error out"=w489:errorcluster)  [unwired: 4 in, 1 out]
                            n442 = Build Path(base path=w490, name or relative path="blank.tif") -> (appended path=w496:path)
                            n443 = local write "CalibInstructions"("Load the fluorophore into the ring(s). You can use the FLUSH and FEED Functions on top or open all valves. Also adjust the microscope for the best acquisition settings. " ("Instructions")) -> ()
                            n444 = Open/Create/Replace File(file path (use dialog)=w496, error in=w489, operation (0:open)=w494) -> (refnum out=w497:refnum<file>, error out=w498:errorcluster)  [unwired: 3 in, 1 out]
                            n445 = local write "CalibImgPath"(w490) -> ()
                            n446 = Close File(refnum=w497, error in=w498) -> (path=w507:path, error out=w500:errorcluster)
                            n447 = call "tiffOpenForWrite.vi"("Path"=w507) -> ("TiffOut"=w510:refnum<k24>)  [unwired: 10 in]
                            n448 = property on="CalibStart" class="Bool (strict)"(error in=w500, "BoolText.Text"="Capture Full Intensity" ("Boolean Text.Text")) -> (error out=w506:errorcluster)  [unwired: 1 in, 1 out]
                            n449 = call "CalibratePositions.vi"("TANGO"=w503, "ANDORExposure"=w509, "CalibStep"=enum16{"Blank", "Full", "Dilution"}."Blank", "error in (no error)"=w506, "Pos List"=w502, ".NET Refnum in"=w510) -> ("error out"=w505:errorcluster, "Image"=w504:T8, ".NET Refnum out"=w499:refnum<k24>)  [unwired: 2 in, 1 out]
                            n450 = call "tiffClose.vi"("Tiff in"=w499) -> ()  [unwired: 10 in, 1 out]
                            n451 = local write "ANDORImage"(w504) -> ()
                          }
                        }
                      }
                      frame "Capture Full Intensity" {
                        n452 = property on="CalibStart" class="Bool (strict)"("BoolText.Text"="Start Dilutions" ("Boolean Text.Text")) -> ()  [unwired: 2 in, 2 out]
                        n453 = local write "CalibInstructions"("Now, switch to the dilution reagent. Make sure it flows through the bypass channel(s) using the FLUSH function." ("Instructions")) -> ()
                        n454 = local read "CalibImgPath"() -> (w518:path)
                        n455 = Build Path(base path=w518, name or relative path="full.tif") -> (appended path=w520:path)
                        n456 = Open/Create/Replace File(file path (use dialog)=w520, error in=w517, operation (0:open)=w512) -> (refnum out=w515:refnum<file>, error out=w516:errorcluster)  [unwired: 3 in, 1 out]
                        n457 = Close File(refnum=w515, error in=w516) -> (path=w514:path, error out=w513:errorcluster)
                        n458 = call "tiffOpenForWrite.vi"("Path"=w514) -> ("TiffOut"=w522:refnum<k24>)  [unwired: 10 in]
                        n459 = call "CalibratePositions.vi"("TANGO"=w524, "ANDORExposure"=w526, "CalibStep"=enum16{"Blank", "Full", "Dilution"}."Full", "error in (no error)"=w513, "Pos List"=w525, ".NET Refnum in"=w522) -> ("error out"=w527:errorcluster, "Image"=w528:T8, ".NET Refnum out"=w521:refnum<k24>)  [unwired: 2 in, 1 out]
                        n460 = call "tiffClose.vi"("Tiff in"=w521) -> ()  [unwired: 10 in, 1 out]
                        n461 = local write "ANDORImage"(w528) -> ()
                      }
                      frame "Start Dilutions" {
                        n462 = local read "CalibImgPath"() -> (w533:path)
                        n463 = Build Path(base path=w533, name or relative path="dilutions.tif") -> (appended path=w540:path)
                        n464 = Open/Create/Replace File(file path (use dialog)=w540, error in=w535, operation (0:open)=w532) -> (refnum out=w537:refnum<file>, error out=w538:errorcluster)  [unwired: 3 in, 1 out]
                        n465 = Close File(refnum=w537, error in=w538) -> (path=w536:path, error out=w534:errorcluster)
                        n466 = call "tiffOpenForWrite.vi"("Path"=w536) -> ("TiffOut"=w541:refnum<k24>)  [unwired: 10 in]
                        n467 = local write "CalibInstructions"("Dilution measurement in progress!" ("Instructions")) -> ()
                        n468 = while {
                          tunnel: w553 -> [w577]
                          shift-right: [w581] -> w544
                          shift-left: w534 -> [w571]
                          shift-right: [w585] -> _
                          shift-left: w552 -> [w588]
                          tunnel: w547 -> [w583]
                          tunnel: w546 -> [w579]
                          tunnel: w545 -> [w578]
                          shift-right: [w570] -> w542
                          shift-left: w541 -> [w569]
                          i -> [w565]
                          stop <- w586 stop-if-true
                          w562 = 10.0 ("y")
                          n469 = Greater Or Equal?(x=w565, y=w562) -> (x >= y?=w573:bool)
                          n470 = local read "ValveFeedRing"() -> (w587:u16)
                          n471 = local read "CalibRestart"() -> (w572:bool)
                          n472 = Add(x=enum16{"Blank", "Full", "Dilution"}."Dilution", y=w565) -> (x+y=w575:i32)
                          n473 = property on="ProgramStop" class="Bool (strict)"() -> ("Value"=w584:bool)  [unwired: 2 in, 2 out]
                          n474 = Compound Arithmetic op=OR(w573, w584, w572, w571) -> (w586:bool)
                          n475 = call "ArdnoDilutionStep.vi"("LINX Resource"=w588, "Single / Multiring?"=w583, "Ring"=w587, "All Rings"=TRUE, "error in (no error)"=w571, "Feed Cycles"="Calib Feed Cycles", "Pump Cycles"="Calib Pump Cycles") -> ("LINX Resource out"=w585:T1, "error out"=w580:errorcluster)  [unwired: 7 in]
                          n476 = Divide(x="Calib Feed Cycles", y=4.0) -> (x/y=w559:dbl)
                          n477 = Divide(x="Calib Pump Cycles", y=5.0 ("Hz")) -> (x/y=w560:dbl)
                          n478 = Add(x=w559, y=w560) -> (x+y=w556:dbl)
                          n479 = Subtract(x=w562, y=w565) -> (x-y=w564:dbl)
                          n480 = call "CalibratePositions.vi"("TANGO"=w579, "ANDORExposure"=w577, "CalibStep"=w575, "error in (no error)"=w580, "Pos List"=w578, ".NET Refnum in"=w569) -> ("error out"=w581:errorcluster, "Elaspsed [ms]"=w557:u32, "Image"=w582:T8, ".NET Refnum out"=w570:refnum<k24>)  [unwired: 2 in]
                          n481 = Divide(x=w557, y=u32 1000) -> (x/y=w555:dbl)
                          n482 = local write "ANDORImage"(w582) -> ()
                          n483 = Add(x=w555, y=w556) -> (x+y=w561:dbl)
                          n484 = Multiply(x=w564, y=w561) -> (x*y=w563:dbl)
                          n485 = local write "CalibRemainingTime"(w563) -> ()
                        }
                        n486 = call "tiffClose.vi"("Tiff in"=w542) -> ()  [unwired: 10 in, 1 out]
                        n487 = call "Get Refresh Ratio from MATLAB"("error in (no error)"=w544) -> ("SinglePumpCycleRefreshRatio"=w550:dbl, "error out"=w548:errorcluster)  [unwired: 16 in, 1 out]
                        n488 = local write "CalibInstructions"("Measurement finished!" ("Instructions")) -> ()
                        n489 = property on="CalibStart" class="Bool (strict)"(error in=w548, "BoolText.Text"="Restart Calibration" ("Boolean Text.Text")) -> (error out=w549:errorcluster)  [unwired: 1 in, 1 out]
                      }
                      frame "Restart Calibration" {
                        n490 = local write "CalibInstructions"("First, capture a blank by adjusting the microscope for a brightfield image of the empty channel. Adjust exposure, objective and filters accordingly. Test it using single images!" ("Instructions")) -> ()
                        n491 = property on="CalibStart" class="Bool (strict)"(error in=w590, "BoolText.Text"="Capture Blank" ("Boolean Text.Text")) -> (error out=w589:errorcluster)  [unwired: 1 in, 1 out]
                      }
                    }
                    n492 = local write "CalibPumpCycleRefreshRatio"(w466) -> ()
                    n493 = property on="CalibStart" class="Bool (strict)"(error in=w467, "DisabledEnum"=T9."Enabled" ("Disabled"), "Value"=FALSE ("Start Pump Calibration")) -> (error out=w475:errorcluster)  [unwired: 1 in, 1 out]
                  }
                  frame "ONERING" {
                    w594 = u16 1 ("Value (Signaling)")
                    w596 = T9."Disabled and Grayed Out" ("Disabled")
                    w595 = FALSE ("ValveFeedRingAll")
                    n494 = property on="ValveFeedRingAll" class="Bool (strict)"("Val(Sgnl)"=w595, "DisabledEnum"=w596) -> ()  [unwired: 2 in, 2 out]
                    n495 = property on="B1" class="Bool (strict)"("Val(Sgnl)"=w595, "DisabledEnum"=w596) -> ()  [unwired: 2 in, 2 out]
                    n496 = property on="B2" class="Bool (strict)"("Val(Sgnl)"=w595, "DisabledEnum"=w596) -> ()  [unwired: 2 in, 2 out]
                    n497 = property on="B3" class="Bool (strict)"("Val(Sgnl)"=w595, "DisabledEnum"=w596) -> ()  [unwired: 2 in, 2 out]
                    n498 = property on="B4" class="Bool (strict)"("Val(Sgnl)"=w595, "DisabledEnum"=w596) -> ()  [unwired: 2 in, 2 out]
                    n499 = property on="A4" class="Bool (strict)"("Val(Sgnl)"=w595, "DisabledEnum"=w596) -> ()  [unwired: 2 in, 2 out]
                    n500 = property on="A5" class="Bool (strict)"("Val(Sgnl)"=w595, "DisabledEnum"=w596) -> ()  [unwired: 2 in, 2 out]
                    n501 = property on="A6" class="Bool (strict)"("Val(Sgnl)"=w595, "DisabledEnum"=w596) -> ()  [unwired: 2 in, 2 out]
                    n502 = property on="A7" class="Bool (strict)"("Val(Sgnl)"=w595, "DisabledEnum"=w596) -> ()  [unwired: 2 in, 2 out]
                    n503 = property on="A8" class="Bool (strict)"("Val(Sgnl)"=w595, "DisabledEnum"=w596) -> ()  [unwired: 2 in, 2 out]
                    n504 = property on="B5" class="Bool (strict)"("Val(Sgnl)"=w595, "DisabledEnum"=w596) -> ()  [unwired: 2 in, 2 out]
                    n505 = property on="B6" class="Bool (strict)"("Val(Sgnl)"=w595, "DisabledEnum"=w596) -> ()  [unwired: 2 in, 2 out]
                    n506 = property on="B7" class="Bool (strict)"("Val(Sgnl)"=w595, "DisabledEnum"=w596) -> ()  [unwired: 2 in, 2 out]
                    n507 = property on="B8" class="Bool (strict)"("Val(Sgnl)"=w595, "DisabledEnum"=w596) -> ()  [unwired: 2 in, 2 out]
                    n508 = property on="ValveFeedReagent" class="DigNum (strict)"("Val(Sgnl)"=w594, "DisabledEnum"=w596) -> ()  [unwired: 2 in, 2 out]
                    n509 = property on="ValveFlushReagent" class="DigNum (strict)"("Val(Sgnl)"=w594, "DisabledEnum"=w596) -> ()  [unwired: 2 in, 2 out]
                  }
                  frame "MULTIRING" {
                    w598 = u16 1 ("Value (Signaling)")
                    w600 = T9."Enabled" ("Disabled")
                    w599 = FALSE ("ValveFeedRingAll")
                    n510 = property on="ValveFeedRingAll" class="Bool (strict)"("Val(Sgnl)"=w599, "DisabledEnum"=w600) -> ()  [unwired: 2 in, 2 out]
                    n511 = property on="B1" class="Bool (strict)"("Val(Sgnl)"=w599, "DisabledEnum"=w600) -> ()  [unwired: 2 in, 2 out]
                    n512 = property on="B2" class="Bool (strict)"("Val(Sgnl)"=w599, "DisabledEnum"=w600) -> ()  [unwired: 2 in, 2 out]
                    n513 = property on="B3" class="Bool (strict)"("Val(Sgnl)"=w599, "DisabledEnum"=w600) -> ()  [unwired: 2 in, 2 out]
                    n514 = property on="B4" class="Bool (strict)"("Val(Sgnl)"=w599, "DisabledEnum"=w600) -> ()  [unwired: 2 in, 2 out]
                    n515 = property on="A4" class="Bool (strict)"("Val(Sgnl)"=w599, "DisabledEnum"=w600) -> ()  [unwired: 2 in, 2 out]
                    n516 = property on="A5" class="Bool (strict)"("Val(Sgnl)"=w599, "DisabledEnum"=w600) -> ()  [unwired: 2 in, 2 out]
                    n517 = property on="A6" class="Bool (strict)"("Val(Sgnl)"=w599, "DisabledEnum"=w600) -> ()  [unwired: 2 in, 2 out]
                    n518 = property on="A7" class="Bool (strict)"("Val(Sgnl)"=w599, "DisabledEnum"=w600) -> ()  [unwired: 2 in, 2 out]
                    n519 = property on="A8" class="Bool (strict)"("Val(Sgnl)"=w599, "DisabledEnum"=w600) -> ()  [unwired: 2 in, 2 out]
                    n520 = property on="B5" class="Bool (strict)"("Val(Sgnl)"=w599, "DisabledEnum"=w600) -> ()  [unwired: 2 in, 2 out]
                    n521 = property on="B6" class="Bool (strict)"("Val(Sgnl)"=w599, "DisabledEnum"=w600) -> ()  [unwired: 2 in, 2 out]
                    n522 = property on="B7" class="Bool (strict)"("Val(Sgnl)"=w599, "DisabledEnum"=w600) -> ()  [unwired: 2 in, 2 out]
                    n523 = property on="B8" class="Bool (strict)"("Val(Sgnl)"=w599, "DisabledEnum"=w600) -> ()  [unwired: 2 in, 2 out]
                    n524 = property on="ValveFeedReagent" class="DigNum (strict)"("Val(Sgnl)"=w598, "DisabledEnum"=w600) -> ()  [unwired: 2 in, 2 out]
                    n525 = property on="ValveFlushReagent" class="DigNum (strict)"("Val(Sgnl)"=w598, "DisabledEnum"=w600) -> ()  [unwired: 2 in, 2 out]
                  }
                }
              }
              n526 = while {
                tunnel: w196 -> [w949]
                tunnel: w167 -> [w947]
                tunnel: w148 -> [w950]
                tunnel: [w943] -> w127
                stop <- w943 stop-if-true
                # "Microsocope Actuation Loop"
                n527 = Dequeue Element(queue=w949, error in (no error)=w950) -> (element=w948:cluster{"Button":string, "Value":dbl}, error out=w944:errorcluster)  [unwired: 1 in, 2 out]
                n528 = Unbundle By Name(w948) -> ("Button"=w945:string, "Value"=w946:dbl)
                n529 = Wait (ms)(milliseconds to wait=u32 50) -> ()  [unwired: 1 out]
                n530 = case shown="\"SAVE SETTINGS\"" w945 {
                  tunnel: w946 -> [w959 w1002 w1008 w1031 _ _ _ _ _ _]
                  tunnel: w944 -> [w957 w1005 w1011 w1034 w1038 w1046 w1051 w1074 w1086 w1127]
                  tunnel: [w952 w995 w1010 w1035 w1036 w1048 w1052 w1061 w1093 w1124] -> w943
                  tunnel: w947 -> [w956 w1006 w1012 w1030 w1037 w1047 _ w1064 _ _]
                  frame "FILTER" {
                    n531 = To Unsigned Long Integer(number=w959) -> (unsigned 32bit integer=w958:u32)
                    n532 = Increment(x=w958) -> (x+1=w953:u32)
                    n533 = case shown="0, Default" w953 {
                      selector: w953 -> [w969 _]
                      tunnel: w957 -> [w973 w991]
                      tunnel: w956 -> [w971 w989]
                      tunnel: [w964 w977] -> w951
                      tunnel: [w968 w987] -> w955
                      tunnel: [w969 u32 6] -> w954
                      frame 0, Default {
                        n534 = call "Set Shutter Status Extended.vi"("VISA Resource Name"=w971, "Shutter Control Number (1)"=1, "Shutter Status (0: Open)"=enum16{"Open", "Close"}."Close", "error in (no error)"=w973) -> ("VISA Resource Name Out"=w968:refnum<visa-resource-name>, "error out"=w965:errorcluster)  [unwired: 10 in]
                        n535 = call "lm Color Enable.vi"("error in (no error)"=w965, "str_State"="ON", "str_Color"="WHITE") -> ("error out"=w963:errorcluster)  [unwired: 6 in, 2 out]
                        n536 = call "lm Get LE State.vi"("error in (no error)"=w963) -> ("error out"=w960:errorcluster, "function return"=w961:i16)  [unwired: 9 in]
                        n537 = Split Number(x=w961) -> (lo(x)=w962:u8)  [unwired: 1 out]
                        n538 = property on="IX81Intensity" class="Slide (strict)"(error in=w960, "Value"=w962) -> (error out=w964:errorcluster)  [unwired: 1 in, 1 out]
                      }
                      frame 7 {
                        n539 = call "Set Shutter Status Extended.vi"("VISA Resource Name"=w989, "Shutter Control Number (1)"=1, "Shutter Status (0: Open)"=enum16{"Open", "Close"}."Open", "error in (no error)"=w991) -> ("VISA Resource Name Out"=w979:refnum<visa-resource-name>, "error out"=w978:errorcluster)  [unwired: 10 in]
                        n540 = call "OlympusQuery.vi"("error in (no error)"=w978, "String"="LMP?", "VISA Resource Name In"=w979) -> ("error out"=w976:errorcluster, "Result"=w984:string, "VISA Resource Name Out"=w987:refnum<visa-resource-name>)  [unwired: 6 in]
                        n541 = Decimal String To Number(string=w984, default (0L)=0.0 ("default (0 I32)")) -> (number=w983:dbl)  [unwired: 1 in, 1 out]
                        n542 = Divide(x=w983, y=1.2 ("x")) -> (x/y=w981:dbl)
                        n543 = property on="IX81Intensity" class="Slide (strict)"("Value"=w981) -> ()  [unwired: 2 in, 2 out]
                        n544 = call "lm Color Enable.vi"("error in (no error)"=w976, "str_State"="OFF", "str_Color"="WHITE") -> ("error out"=w977:errorcluster)  [unwired: 6 in, 2 out]
                      }
                    }
                    n545 = call "Select Filter Wheel.vi"("error in (no error)"=w951, "Filter Wheel Position (1)"=w954, "VISA Resource Name"=w955) -> ("error out"=w952:errorcluster)  [unwired: 7 in, 1 out]
                  }
                  frame "FOCUS" {
                    n546 = call "Move Focusing Unit.vi"("VISA Resource Name"=w1006, "Device Number (1)"=2, "Direction (1: Down)"=enum16{"Up", "Down", "Abs"}."Abs", "Step (0.0 um)"=w1002, "error in (no error)"=w1005) -> ("VISA Resource Name Out"=w997:refnum<visa-resource-name>, "error out"=w996:errorcluster)  [unwired: 9 in]
                    n547 = call "OlympusQuery.vi"("error in (no error)"=w996, "Device Number\n(1: -Condensor\n     - Objective\n     - Lamp\n     - Shutter\n2: - Z-Motion\n   - Autofocus)"=2 ("Device Number\n(1: -Condensor\n     - Objective\n     - Lamp\n     - Shutter\n2: - Z-Motion\n   - Autofocus)"), "String"="POS?", "VISA Resource Name In"=w997) -> ("error out"=w995:errorcluster, "Result"=w1001:string)  [unwired: 5 in, 1 out]
                    n548 = Decimal String To Number(string=w1001, default (0L)=0.0 ("default (0 I32)")) -> (number=w994:dbl)  [unwired: 1 in, 1 out]
                    n549 = Divide(x=w994, y=1000.0) -> (x/y=w993:dbl)
                    n550 = local write "IX81Focus"(w993) -> ()
                  }
                  frame "INTENSITY" {
                    n551 = property on="IX81Filter" class="Ring (strict)"() -> ("RingText.Text"=w1009:string)  [unwired: 2 in, 2 out]
                    n552 = Round To Nearest(number=w1008) -> (nearest integer value=w1007:dbl)
                    n553 = case shown="\"GFP\", Default" w1009 {
                      tunnel: w1007 -> [w1023 w1029]
                      tunnel: w1012 -> [_ w1027]
                      tunnel: w1011 -> [w1016 w1025]
                      tunnel: [w1014 w1024] -> w1010
                      frame "GFP", Default {
                        n554 = Greater Than 0?(x=w1023) -> (x > 0?=w1018:bool)
                        n555 = Boolean To (0,1)(Boolean=w1018) -> (0, 1=w1020:i16)
                        n556 = Index Array(array=string[] ["OFF", "ON"], index=w1020) -> (element=w1019:string)
                        n557 = call "lm Color Enable.vi"("error in (no error)"=w1016, "str_State"=w1019, "str_Color"="WHITE") -> ("error out"=w1015:errorcluster, "str_Color out"=w1013:string)  [unwired: 6 in, 1 out]
                        n558 = Number To Decimal String(number=w1023) -> (decimal integer string=w1022:string)  [unwired: 1 in]
                        n559 = call "lm Color Level.vi"("error in (no error)"=w1015, "str_Level"=w1022, "str_Color"=w1013) -> ("error out"=w1014:errorcluster)  [unwired: 6 in, 2 out]
                      }
                      frame "Bright Field" {
                        n560 = Multiply(x=w1029, y=0.12) -> (x*y=w1026:dbl)
                        n561 = call "Configure Lamp.vi"("VISA Resource Name"=w1027, "Lamp Intensity (1.0 V)"=w1026, "error in (no error)"=w1025) -> ("error out"=w1024:errorcluster)  [unwired: 11 in, 1 out]
                      }
                    }
                  }
                  frame "OBJECTIVE" {
                    n562 = To Unsigned Long Integer(number=w1031) -> (unsigned 32bit integer=w1033:u32)
                    n563 = Increment(x=w1033) -> (x+1=w1032:u32)
                    n564 = call "Set Active Objective.vi"("error in (no error)"=w1034, "Objective Number (1)"=w1032, "VISA Resource Name"=w1030) -> ("error out"=w1035:errorcluster)  [unwired: 7 in, 1 out]
                  }
                  frame "FOCUSUPDATE" {
                    n565 = call "OlympusQuery.vi"("error in (no error)"=w1038, "Device Number\n(1: -Condensor\n     - Objective\n     - Lamp\n     - Shutter\n2: - Z-Motion\n   - Autofocus)"=2 ("Device Number\n(1: -Condensor\n     - Objective\n     - Lamp\n     - Shutter\n2: - Z-Motion\n   - Autofocus)"), "String"="POS?", "VISA Resource Name In"=w1037) -> ("error out"=w1036:errorcluster, "Result"=w1043:string)  [unwired: 5 in, 1 out]
                    n566 = Decimal String To Number(string=w1043, default (0L)=0.0 ("default (0 I32)")) -> (number=w1044:dbl)  [unwired: 1 in, 1 out]
                    n567 = Divide(x=w1044, y=1000.0) -> (x/y=w1045:dbl)
                    n568 = local write "IX81Focus"(w1045) -> ()
                  }
                  frame "PRISM" {
                    n569 = local read "IX81Prism"() -> (w1049:u16)
                    n570 = To Unsigned Long Integer(number=w1049) -> (unsigned 32bit integer=w1050:u32)
                    n571 = call "Select Prism.vi"("error in (no error)"=w1046, "Prism Position (0: Bi)"=w1050, "VISA Resource Name"=w1047) -> ("error out"=w1048:errorcluster)  [unwired: 7 in, 1 out]
                  }
                  frame "", Default {
                    n572 = Merge Errors(errorcluster {"status"=FALSE, "code"=9999, "source"="Unknown Element in the queue"} ("error constant"), w1051) -> (w1052:errorcluster)
                  }
                  frame "APPEND SETTINGS" {
                    n573 = call "OlympusQuery.vi"("error in (no error)"=w1074, "String"="MU?", "VISA Resource Name In"=w1064) -> ("error out"=w1082:errorcluster, "Result"=w1077:string, "VISA Resource Name Out"=w1081:refnum<visa-resource-name>)  [unwired: 6 in]
                    n574 = Decimal String To Number(string=w1077) -> (number=w1078:i32)  [unwired: 2 in, 1 out]
                    n575 = local read "IX81Intensity"() -> (w1055:dbl)
                    n576 = Decrement(x=w1078) -> (x-1=w1065:i32)
                    n577 = call "OlympusQuery.vi"("error in (no error)"=w1082, "String"="OB?", "VISA Resource Name In"=w1081) -> ("error out"=w1056:errorcluster, "Result"=w1079:string)  [unwired: 6 in, 1 out]
                    n578 = property on="IX81Filter" class="Ring (strict)"(error in=w1056) -> (error out=w1062:errorcluster, "Strings []"=w1073:string[])  [unwired: 1 in, 1 out]
                    n579 = Decimal String To Number(string=w1079) -> (number=w1080:i32)  [unwired: 2 in, 1 out]
                    n580 = Number To Fractional String(number=w1055, precision (6)=i16 1) -> (F-format string=w1063:string)  [unwired: 2 in]
                    n581 = Index Array(array=w1073, index=w1065) -> (element=w1067:string)
                    n582 = property on="IX81Objective" class="Enum (strict)"() -> ("Strings []"=w1071:string[])  [unwired: 2 in, 2 out]
                    n583 = local read "ANDORExposure"() -> (w1057:sgl)
                    n584 = Decrement(x=w1080) -> (x-1=w1072:i32)
                    n585 = property on="IX81Prism" class="Ring (strict)"() -> ("RingText.Text"=w1059:string)  [unwired: 2 in, 2 out]
                    n586 = Index Array(array=w1071, index=w1072) -> (element=w1070:string)
                    n587 = Number To Decimal String(number=w1057) -> (decimal integer string=w1058:string)  [unwired: 1 in]
                    n588 = property on="IX81Settings" class="MCListbox (strict)"() -> ("ItemNames"=w1068:string[][])  [unwired: 2 in, 2 out]
                    n589 = Build Array(w1070, w1067, w1059, w1063, w1058) -> (w1069:string[])
                    n590 = property on="IX81SettingsAppend" class="Bool (strict)"(error in=w1062, "Value"=FALSE ("Clear Microscope Settings")) -> (error out=w1061:errorcluster)  [unwired: 1 in, 1 out]
                    n591 = Build Array (concatenate)(w1068, w1069) -> (w1066:string[][])
                    n592 = property on="IX81Settings" class="MCListbox (strict)"("ItemNames"=w1066) -> ()  [unwired: 2 in, 2 out]
                  }
                  frame "SAVE SETTINGS" {
                    n593 = call "File Dialog2"("start path"=path "../../Config_Files", "error in"=w1086, "pattern (all files)"="*.xml", "pattern label"="Configuration XML") -> ("selected path"=w1088:path, "cancelled"=w1084:bool, "error out"=w1089:errorcluster)  [unwired: 8 in, 1 out]
                    n594 = case shown="True" w1084 {
                      tunnel: w1089 -> [w1118 w1122]
                      tunnel: w1088 -> [w1117 _]
                      tunnel: [w1111 w1122] -> w1087
                      tunnel: T11."replace or create with confirmation" ("operation (0:open)") -> [w1108 _]
                      frame False {
                        n595 = Open/Create/Replace File(file path (use dialog)=w1117, error in=w1118, operation (0:open)=w1108) -> (refnum out=w1113:refnum<file>, error out=w1116:errorcluster)  [unwired: 3 in, 1 out]
                        n596 = property on="IX81Settings" class="MCListbox (strict)"() -> ("ItemNames"=w1121:string[][])  [unwired: 2 in, 2 out]
                        n597 = Set File Size(4:w1116, 6:i64 0 ("size (in bytes)"), 7:w1113) -> (0:w1110:errorcluster, 3:w1114:refnum<file>)
                        n598 = Transpose 2D Array(2D array=w1121) -> (transposed array=w1107:string[][])
                        n599 = call "ConfigFlattenMicroscopeToXML.vi"("error in (no error)"=w1110, "MicroscopeArray"=w1107) -> ("error out"=w1109:errorcluster, "MicrosocopeXML"=w1115:string)  [unwired: 8 in]
                        n600 = Concatenate Strings("<" ("string"), "Loop" ("string"), ">" ("string"), "\r\n") -> (w1101:string)
                        n601 = Concatenate Strings("</" ("string"), "Loop" ("string"), ">" ("string"), "\r\n") -> (w1096:string)
                        n602 = Concatenate Strings("<?xml version=\"1.0\" encoding=\"UTF-8\" standalone=\"no\" ?>\n<Measurement xmlns:xsi=\"http://www.w3.org/2001/XMLSchema-instance\" xsi:noNamespaceSchemaLocation=\"C:\\Users\\e14user\\Documents\\LabVIEW software\\GitRepo\\lib\\Config\\validator.xsd\">", w1101, w1115, w1096, "</Measurement>" ("string")) -> (w1106:string)
                        n603 = Write to Text File(file (use dialog)=w1114, text=w1106, error in=w1109) -> (refnum out=w1120:refnum<file>, error out=w1119:errorcluster)  [unwired: 1 in, 1 out]
                        n604 = Close File(refnum=w1120, error in=w1119) -> (error out=w1111:errorcluster)  [unwired: 1 out]
                      }
                      frame True {
                      }
                    }
                    n605 = property on="IX81SettingsSave" class="Bool (strict)"(error in=w1087, "Value"=FALSE ("Clear Microscope Settings")) -> (error out=w1093:errorcluster)  [unwired: 1 in, 1 out]
                  }
                  frame "CLEAR SETTINGS" {
                    n606 = property on="IX81Settings" class="MCListbox (strict)"(error in=w1127) -> (error out=w1126:errorcluster, "ItemNames"=w1133:string[][])  [unwired: 1 in, 1 out]
                    n607 = Array Size(array=w1133) -> (size(s)=w1132:i32[])
                    n608 = Index Array(array=w1132, index=0) -> (element=w1131:i32)
                    n609 = Decrement(x=w1131) -> (x-1=w1128:i32)
                    n610 = case shown="1, Default" w1128 {
                      selector: w1128 -> [_ w1135]
                      tunnel: w1133 -> [w1134 w1137]
                      tunnel: [w1134 w1136] -> w1129
                      frame -1 {
                      }
                      frame 1, Default {
                        n611 = Delete From Array(array=w1137, index (row)=w1135) -> (array with subset deleted=w1136:string[][])  [unwired: 2 in, 1 out]
                      }
                    }
                    n612 = property on="IX81Settings" class="MCListbox (strict)"(error in=w1126, "ItemNames"=w1129) -> (error out=w1125:errorcluster)  [unwired: 1 in, 1 out]
                    n613 = property on="IX81SettingsClear" class="Bool (strict)"(error in=w1125, "Value"=FALSE ("Append Current Settings")) -> (error out=w1124:errorcluster)  [unwired: 1 in, 1 out]
                  }
                }
              }
              n614 = call <vilib>:"Clear Errors.vi"("error in (no error)"=w133, "specific error code to clear (0: all)"=1122) -> ("error out"=w134:errorcluster)  [unwired: 4 in, 1 out]
              n615 = call <vilib>:"Clear Errors.vi"("error in (no error)"=w127, "specific error code to clear (0: all)"=1) -> ("error out"=w128:errorcluster)  [unwired: 4 in, 1 out]
              n616 = call <vilib>:"Clear Errors.vi"("error in (no error)"=w144, "specific error code to clear (0: all)"=w136) -> ("error out"=w137:errorcluster)  [unwired: 4 in, 1 out]
              n617 = call <vilib>:"Clear Errors.vi"("error in (no error)"=w130, "specific error code to clear (0: all)"=1122) -> ("error out"=w131:errorcluster)  [unwired: 4 in, 1 out]
              n618 = Flush Queue(queue=w158, error in (no error)=w155) -> (queue out=w159:refnum<queue>, error out=w157:errorcluster)  [unwired: 1 out]
              n619 = Release Queue(queue=w159, force destroy? (F)=TRUE, error in (no error)=w157) -> (error out=w174:errorcluster)  [unwired: 2 out]
              n620 = Merge Errors(w174, w134) -> (w141:errorcluster)
              n621 = Flush Queue(queue=w204, error in (no error)=w153) -> (queue out=w202:refnum<queue>, error out=w203:errorcluster)  [unwired: 1 out]
              n622 = Release Queue(queue=w202, force destroy? (F)=TRUE, error in (no error)=w203) -> (error out=w173:errorcluster)  [unwired: 2 out]
              n623 = Merge Errors(w128, w173) -> (w138:errorcluster)
              n624 = call "IMAQ Dispose"("All Images? (No)"=TRUE, "Image"=w161, "error in (no error)"=w137) -> ("error out"=w142:errorcluster)  [unwired: 3 in]
              n625 = Release Queue(queue=w156, force destroy? (F)=TRUE, error in (no error)=w154) -> (error out=w175:errorcluster)  [unwired: 2 out]
              n626 = Merge Errors(w142, w175) -> (w143:errorcluster)
              n627 = Flush Queue(queue=w198, error in (no error)=w139) -> (queue out=w166:refnum<queue>, error out=w165:errorcluster)  [unwired: 1 out]
              n628 = Release Queue(queue=w166, force destroy? (F)=TRUE, error in (no error)=w165) -> (error out=w172:errorcluster)  [unwired: 2 out]
              n629 = Merge Errors(w172, w131) -> (w140:errorcluster)
              n630 = Merge Errors(w143, w178, w141, w176, w140, w138) -> (w123:errorcluster)
              n631 = local read "ProgramCreate"() -> (w125:bool)
              n632 = local read "ProgramRun"() -> (w124:bool)
              n633 = local read "ProgramStop"() -> (w147:bool)
              n634 = Compound Arithmetic op=OR(w123, w124, w125, w147) -> (w126:bool)
            }
          }
          frame #1 {
            n635 = while {
              tunnel: [w1554] -> w1243
              tunnel: [w1553] -> w1244
              tunnel: [w1552] -> w1245
              tunnel: [w1551] -> w1246
              tunnel: [w1550] -> w1242
              tunnel: [w1549] -> w1247
              tunnel: [w1548] -> w1248
              tunnel: [w1547] -> w1249
              tunnel: [w1546] -> w1250
              stop <- w1556 stop-if-true
              # "Continuous Program Initialization"
              n636 = event shown="[2] \"ProgramCreate\": Value Change" {
                selector: _ -> [_ _ _]
                dyn-events: _ -> [_ _ _]
                timeout: 1 -> [_ _ _]
                tunnel: [FALSE ("StartProgram") w1568 w1596] -> w1554
                tunnel: [_ w1567 _] -> w1553
                tunnel: [_ w1566 _] -> w1552
                tunnel: [_ w1565 _] -> w1551
                tunnel: [errorcluster {"status"=FALSE, "code"=0, "source"=""} ("error out") w1564 errorcluster {"status"=FALSE, "code"=0, "source"=""} ("error out")] -> w1550
                tunnel: [_ w1563 _] -> w1549
                tunnel: [_ w1562 _] -> w1548
                tunnel: [_ w1561 _] -> w1547
                tunnel: [_ w1560 _] -> w1546
                event Timeout {
                  n637 = event-data() -> ()  [unwired: 1 in, 3 out]
                }
                event "ProgramRun": Value Change {
                  n638 = event-data() -> ("NewVal"=w1569:bool)  [unwired: 1 in, 5 out]
                  n639 = case shown="True" w1569 {
                    tunnel: [w1586 FALSE ("StartProgram")] -> w1568
                    tunnel: [w1585 _] -> w1567
                    tunnel: [w1584 _] -> w1566
                    tunnel: [w1583 _] -> w1565
                    tunnel: [w1582 _] -> w1564
                    tunnel: [w1581 _] -> w1563
                    tunnel: [w1580 _] -> w1562
                    tunnel: [w1579 _] -> w1561
                    tunnel: [w1578 _] -> w1560
                    frame True {
                      w1574 = T9."Enabled" ("Disabled")
                      n640 = local write "ProgramStatusInfo"("Parsing Files and preparing queue" ("Info")) -> ()
                      n641 = property on="Pane" class="Pane"() -> (error out=w1576:errorcluster, "Controls[]"=w1575:refnum<vi>[])  [unwired: 2 in, 1 out]
                      n642 = for {
                        tunnel: w1575 -> [w1590] mode=indexing
                        tunnel: T9."Disabled and Grayed Out" ("Disabled") -> [w1589]
                        shift-right: [w1587] -> w1577
                        shift-left: w1576 -> [w1588]
                        n643 = property class="Ctl"(reference=w1590, error in=w1588, "DisabledEnum"=w1589) -> (error out=w1587:errorcluster)  [unwired: 1 out]
                      }
                      n644 = property on="ProgramStop" class="Bool (strict)"(error in=w1577, "DisabledEnum"=w1574) -> (error out=w1570:errorcluster)  [unwired: 1 in, 1 out]
                      n645 = property on="ANDORImage" class="ImageControl"(error in=w1570, "DisabledEnum"=w1574) -> (error out=w1571:errorcluster)  [unwired: 1 in, 1 out]
                      n646 = call "ContinousLoopMain.vi"("error in"=w1571) -> ("SaveDir"=w1579:path, "File Prefix"=w1578:string, "Total Duration"=w1581:timestamp, "Interval"=w1580:timestamp, "queue out"=w1583:refnum<queue>, "Microscope"=w1584:T15, "StartProgram"=w1586:bool, "Positions"=w1585:dbl[][], "error out"=w1582:errorcluster)  [unwired: 6 in]
                    }
                    frame False, Default {
                      n647 = property on="Pane" class="Pane"() -> ("Controls[]"=w1593:refnum<vi>[])  [unwired: 2 in, 2 out]
                      n648 = for {
                        tunnel: w1593 -> [w1595] mode=indexing
                        tunnel: T9."Enabled" ("Disabled") -> [w1594]
                        n649 = property class="Ctl"(reference=w1595, "DisabledEnum"=w1594) -> ()  [unwired: 1 in, 2 out]
                      }
                    }
                  }
                }
                event "ProgramCreate": Value Change {
                  n650 = event-data() -> ()  [unwired: 1 in, 6 out]
                  n651 = flat-sequence {
                    tunnel: [w1598] -> w1596
                    frame #0 {
                      # "Create Program"
                      n652 = local read "CalibPumpCycleRefreshRatio"() -> (w1599:dbl)
                      n653 = call "ConfigCreateProgram.vi"("singlePumpCycleRefreshRatio"=w1599) -> ("stop 2"=w1598:bool)  [unwired: 10 in]
                    }
                    frame #1 {
                      # "Reset Button on Finish"
                      n654 = property on="ProgramCreate" class="Bool (strict)"("Value"=FALSE ("CreateProgram")) -> ()  [unwired: 2 in, 2 out]
                    }
                  }
                }
              }
              n655 = local read "ProgramStop"() -> (w1555:bool)
              n656 = Or(x=w1554, y=w1555) -> (x .or. y?=w1556:bool)
            }
            n657 = case shown="True" w1243 {
              tunnel: w1244 -> [_ w1272]
              tunnel: w1245 -> [_ w1271]
              tunnel: w1246 -> [_ w1273]
              tunnel: w1242 -> [w1251 w1274]
              tunnel: w1247 -> [_ w1259]
              tunnel: w1248 -> [_ w1261]
              tunnel: w1249 -> [_ w1279]
              tunnel: w1250 -> [_ w1278]
              tunnel: [w1251 w1277] -> _
              frame False {
              }
              frame True {
                # "Program Execution"
                n658 = To Double Precision Float(number=w1259) -> (double precision float=w1260:dbl)
                n659 = To Double Precision Float(number=w1261) -> (double precision float=w1262:dbl)
                n660 = Negate(x=w1260) -> (-x=w1258:dbl)
                n661 = local read "IX 81 Port"() -> (w1276:refnum<visa-resource-name>)
                n662 = local write "ProgramStatusInfo"("Initializing Program" ("Info")) -> ()
                n663 = call "Select Prism.vi"("error in (no error)"=w1274, "Prism Position (0: Bi)"=enum16{"Bi", "Side"}."Side", "VISA Resource Name"=w1276) -> ("error out"=w1265:errorcluster, "VISA Resource Name Out"=w1267:refnum<visa-resource-name>)  [unwired: 7 in]
                n664 = call "Set Shutter Status Extended.vi"("VISA Resource Name"=w1267, "Shutter Status (0: Open)"=enum16{"Open", "Close"}."Close", "error in (no error)"=w1265) -> ("VISA Resource Name Out"=w1266:refnum<visa-resource-name>, "error out"=w1264:errorcluster)  [unwired: 11 in]
                n665 = for {
                  tunnel: w1271 -> [w1288] mode=indexing
                  shift-right: [w1280] -> w1270
                  shift-left: w1266 -> [w1283]
                  shift-right: [w1281] -> w1256
                  shift-left: w1264 -> [w1282]
                  n666 = Unbundle By Name(w1288) -> ("Filter"=w1285:string, "Intensity"=w1284:dbl)
                  n667 = Equal?(x="BF", y=w1285) -> (x = y?=w1287:bool)
                  n668 = case shown="True" w1287 {
                    tunnel: w1284 -> [_ w1298]
                    tunnel: w1283 -> [w1290 w1297]
                    tunnel: w1282 -> [w1289 w1296]
                    tunnel: [w1289 w1295] -> w1281
                    tunnel: [w1290 w1294] -> w1280
                    frame False {
                    }
                    frame True {
                      n669 = Multiply(x=w1298, y=0.12) -> (x*y=w1292:dbl)
                      n670 = call "Configure Lamp.vi"("VISA Resource Name"=w1297, "Lamp Intensity (1.0 V)"=w1292, "error in (no error)"=w1296) -> ("VISA Resource Name Out"=w1294:refnum<visa-resource-name>, "error out"=w1295:errorcluster)  [unwired: 11 in]
                      n671 = Wait (ms)(milliseconds to wait=u32 30000) -> ()  [unwired: 1 out]
                    }
                  }
                }
                n672 = Get Date/Time In Seconds() -> (seconds since 1Jan1904=w1252:timestamp)
                n673 = Negate(x=w1262) -> (-x=w1253:dbl)
                n674 = property on="ProgramStatusInfo" class="Str"(error in=w1256, "Text.Text"="Initialization Finished") -> (error out=w1255:errorcluster)  [unwired: 1 in, 1 out]
                n675 = Add(x=w1258, y=w1252) -> (x+y=w1268:timestamp)
                n676 = Add(x=w1252, y=w1253) -> (x+y=w1269:timestamp)
                n677 = while {
                  tunnel: w1279 -> [w1326]
                  tunnel: w1278 -> [w1323]
                  shift-right: [w1311] -> w1277
                  shift-left: w1255 -> [w1321]
                  shift-right: [w1310] -> _
                  shift-left: w1270 -> [w1305]
                  shift-right: [w1319] -> _
                  shift-left: w1273 -> [w1318]
                  tunnel: w1272 -> [w1313]
                  tunnel: w1271 -> [w1312]
                  tunnel: w1253 -> [w1303]
                  shift-right: [w1302] -> _
                  shift-left: w1269 -> [w1304]
                  tunnel: w1268 -> [w1300]
                  stop <- w1308 stop-if-true
                  # "Executing Program Loop"
                  n678 = Get Date/Time In Seconds() -> (seconds since 1Jan1904=w1301:timestamp)
                  n679 = Greater Or Equal?(x=w1301, y=w1300) -> (x >= y?=w1327:bool)
                  n680 = property on="ProgramStop" class="Bool (strict)"() -> ("Value"=w1299:bool)  [unwired: 2 in, 2 out]
                  n681 = Format Date/Time String(time format string (%c)="%y%m%d_%H_%M_%S_", seconds (now)=w1301) -> (date/time string=w1324:string)  [unwired: 1 in]
                  n682 = Or(x=w1327, y=w1299) -> (x .or. y?=w1328:bool)
                  n683 = Concatenate Strings(w1324, w1323) -> (w1322:string)
                  n684 = Dequeue Element(queue=w1318, error in (no error)=w1321) -> (queue out=w1319:refnum<queue>, element=w1320:T16, timed out?=w1307:bool, error out=w1309:errorcluster)  [unwired: 1 in]
                  n685 = Unbundle By Name(w1320) -> ("Step Name"=w1317:string, "Time"=w1316:dbl, "Param 1"=w1306:dbl, "Param 2"=w1315:i32)
                  n686 = Or(x=w1307, y=w1328) -> (x .or. y?=w1308:bool)
                  n687 = Build Path(base path=w1326, name or relative path=w1322) -> (appended path=w1314:path)
                  n688 = case shown="\"PUMP\"" w1317 {
                    tunnel: w1316 -> [_ w1476 w1489 _ _ w1521]
                    tunnel: w1306 -> [_ _ w1491 _ w1507 w1526]
                    tunnel: w1315 -> [_ _ _ _ _ _]
                    tunnel: w1309 -> [w1338 w1473 w1496 w1498 w1505 w1529]
                    tunnel: w1314 -> [w1344 _ _ _ _ _]
                    tunnel: w1313 -> [w1342 _ _ _ _ _]
                    tunnel: w1312 -> [w1331 _ _ _ _ _]
                    tunnel: w1305 -> [w1341 w1472 w1490 w1497 w1515 w1527]
                    tunnel: [w1340 w1470 w1492 w1498 w1501 w1525] -> w1311
                    tunnel: [w1339 w1472 w1490 w1497 w1515 w1527] -> w1310
                    tunnel: w1304 -> [w1336 w1471 w1488 w1499 w1500 _]
                    tunnel: w1303 -> [w1333 _ _ _ _ _]
                    tunnel: [w1332 w1471 w1488 w1499 w1500 _] -> w1302
                    frame "ACQUIRE" {
                      n689 = Get Date/Time In Seconds() -> (seconds since 1Jan1904=w1334:timestamp)
                      n690 = Array Size(array=w1342) -> (size(s)=w1345:i32[])
                      n691 = Less?(x=w1334, y=w1336) -> (x < y?=w1337:bool)
                      n692 = Subtract(x=w1334, y=w1336) -> (x-y=w1335:dbl)
                      "Program Timing Offset" <- w1335
                      n693 = Array Size(array=w1331) -> (size(s)=w1330:i32)
                      n694 = Index Array(array=w1345, index=0) -> (element=w1329:i32)
                      n695 = Multiply(x=w1330, y=w1329) -> (x*y=w1346:i32)
                      n696 = call "tiffOpenForWrite.vi"("Path"=w1344) -> ("TiffOut"=w1347:refnum<k24>)  [unwired: 10 in]
                      n697 = case shown="True" w1337 {
                        tunnel: w1335 -> [_ w1361]
                        tunnel: w1334 -> [w1354 w1356]
                        tunnel: w1333 -> [w1355 w1357]
                        tunnel: [w1353 w1358] -> w1332
                        frame False {
                          n698 = Add(x=w1354, y=w1355) -> (x+y=w1353:timestamp)
                        }
                        frame True {
                          n699 = Add(x=w1356, y=w1357) -> (x+y=w1358:timestamp)
                          n700 = Multiply(x=1000.0, y=w1361) -> (x*y=w1359:dbl)
                          n701 = Wait (ms)(milliseconds to wait=w1359) -> ()  [unwired: 1 out]
                        }
                      }
                      n702 = for {
                        tunnel: w1342 -> [w1375] mode=indexing
                        tunnel: w1331 -> [w1386]
                        tunnel: w1346 -> [w1363]
                        shift-right: [w1388] -> w1348
                        shift-left: w1347 -> [w1362]
                        shift-right: [w1368] -> w1340
                        shift-left: w1338 -> [w1373]
                        tunnel: [w1367] -> w1349
                        shift-right: [w1365] -> w1339
                        shift-left: w1341 -> [w1366]
                        i -> [w1385]
                        stop <- w1364 stop-if-true
                        # "TANGO\n drive to positions"
                        # "Drive to all positions"
                        n703 = Index Array(array=w1375, index=0) -> (element=w1380:dbl)
                        n704 = Index Array(array=w1375, index=1) -> (element=w1378:dbl)
                        n705 = Index Array(array=w1375, index=2) -> (element=w1374:dbl)
                        n706 = local read "TANGO"() -> (w1377:i32)
                        n707 = call <userlib>:"LSX Move Abs.vi"("error in (no error)"=w1373, "dY"=w1378, "dX"=w1380, "lLSID"=w1377) -> ("error out"=w1372:errorcluster)  [unwired: 6 in, 1 out]
                        n708 = call "Move Focusing Unit.vi"("VISA Resource Name"=w1366, "Device Number (1)"=2, "Direction (1: Down)"=enum16{"Up", "Down", "Abs"}."Abs", "Step (0.0 um)"=w1374, "error in (no error)"=w1373) -> ("VISA Resource Name Out"=w1370:refnum<visa-resource-name>, "error out"=w1371:errorcluster)  [unwired: 9 in]
                        n709 = Merge Errors(w1372, w1371) -> (w1369:errorcluster)
                        n710 = Number To Decimal String(number=w1385) -> (decimal integer string=w1387:string)  [unwired: 1 in]
                        n711 = Increment(x=w1385) -> (x+1=w1384:i32)
                        n712 = for {
                          shift-right: [w1389] -> w1388
                          shift-left: _ -> [_]
                          tunnel: w1387 -> [w1416]
                          tunnel: w1386 -> [w1418] mode=indexing
                          tunnel: w1384 -> [w1413]
                          shift-right: [w1397] -> w1368
                          shift-left: w1369 -> [w1408]
                          tunnel: [w1390] -> w1367
                          shift-right: [w1398] -> w1365
                          shift-left: w1370 -> [w1411]
                          tunnel: w1363 -> [w1395]
                          tunnel: w1362 -> [w1391]
                          i -> [w1414]
                          stop <- w1396 stop-if-true
                          # "Loop over all images"
                          n713 = Unbundle By Name(w1418) -> ("Objective"=w1410:i32, "Filter"=w1403:string, "Intensity"=w1401:dbl, "Exposure"=w1393:i32)  [unwired: 1 out]
                          n714 = case shown="100" w1410 {
                            tunnel: [2 3 4 5 1] -> w1409
                            frame 10 {
                            }
                            frame 20 {
                            }
                            frame 40 {
                            }
                            frame 100 {
                            }
                            frame 4, Default {
                            }
                          }
                          n715 = Increment(x=w1414) -> (x+1=w1412:i32)
                          n716 = Add(x=w1412, y=w1413) -> (x+y=w1415:i32)
                          n717 = Decrement(x=w1415) -> (x-1=w1394:i32)
                          n718 = call "Set Active Objective.vi"("error in (no error)"=w1408, "Objective Number (1)"=w1409, "VISA Resource Name"=w1411) -> ("error out"=w1405:errorcluster, "VISA Resource Name Out"=w1406:refnum<visa-resource-name>)  [unwired: 7 in]
                          n719 = property on="IX81Filter" class="Ring (strict)"() -> ("Strings []"=w1404:string[])  [unwired: 2 in, 2 out]
                          n720 = Number To Decimal String(number=w1414) -> (decimal integer string=w1417:string)  [unwired: 1 in]
                          n721 = Search 1D Array(1D array=w1404, element=w1403) -> (index of element=w1402:i32)  [unwired: 1 in]
                          n722 = Increment(x=w1402) -> (x+1=w1407:i32)
                          n723 = Concatenate Strings(w1416, w1417, w1403) -> (w1392:string)
                          n724 = call "Select Filter Wheel.vi"("error in (no error)"=w1405, "Filter Wheel Position (1)"=w1407, "VISA Resource Name"=w1406) -> ("error out"=w1400:errorcluster, "VISA Resource Name Out"=w1399:refnum<visa-resource-name>)  [unwired: 7 in]
                          n725 = case shown="0, Default" w1402 {
                            tunnel: w1401 -> [w1441 _]
                            tunnel: w1400 -> [w1439 w1462]
                            tunnel: w1399 -> [w1440 w1463]
                            tunnel: [w1437 w1452] -> w1398
                            tunnel: [w1438 w1442] -> w1397
                            tunnel: w1395 -> [w1435 w1460]
                            tunnel: w1394 -> [w1434 w1459]
                            tunnel: w1393 -> [w1433 w1458]
                            tunnel: w1392 -> [w1432 w1457]
                            tunnel: w1391 -> [w1431 w1456]
                            tunnel: [w1430 w1455] -> w1390
                            tunnel: [w1429 w1454] -> w1389
                            frame 0, Default {
                              n726 = call "Set Shutter Status Extended.vi"("VISA Resource Name"=w1440, "Shutter Status (0: Open)"=enum16{"Open", "Close"}."Close", "error in (no error)"=w1439) -> ("VISA Resource Name Out"=w1437:refnum<visa-resource-name>, "error out"=w1422:errorcluster)  [unwired: 11 in]
                              n727 = call "lm Color Enable.vi"("error in (no error)"=w1422, "str_State"="ON", "str_Color"="WHITE") -> ("error out"=w1423:errorcluster, "str_Color out"=w1421:string)  [unwired: 6 in, 1 out]
                              n728 = Number To Decimal String(number=w1441) -> (decimal integer string=w1427:string)  [unwired: 1 in]
                              n729 = call "lm Color Level.vi"("error in (no error)"=w1423, "str_Level"=w1427, "str_Color"=w1421) -> ("error out"=w1436:errorcluster)  [unwired: 6 in, 2 out]
                              n730 = call "AndorAcqSingleImgToTiffStack.vi"("Image Nr"=w1434, "Total Images"=w1435, "error in (no error)"=w1436, "Exposure"=w1433, "Image Name"=w1432, "TiffHandle IN"=w1431) -> ("error out"=w1428:errorcluster, "Image"=w1430:T8, "TiffOut"=w1429:refnum<k24>)  [unwired: 3 in]
                              n731 = call "lm Color Enable.vi"("error in (no error)"=w1428, "str_State"="OFF", "str_Color"="WHITE") -> ("error out"=w1438:errorcluster)  [unwired: 6 in, 2 out]
                            }
                            frame 5 {
                              n732 = call "Set Shutter Status Extended.vi"("VISA Resource Name"=w1463, "Shutter Status (0: Open)"=enum16{"Open", "Close"}."Open", "error in (no error)"=w1462) -> ("VISA Resource Name Out"=w1443:refnum<visa-resource-name>, "error out"=w1445:errorcluster)  [unwired: 11 in]
                              n733 = call "lm Color Enable.vi"("error in (no error)"=w1445, "str_State"="OFF", "str_Color"="WHITE") -> ("error out"=w1446:errorcluster, "str_Color out"=w1447:string)  [unwired: 6 in, 1 out]
                              n734 = call "lm Color Level.vi"("error in (no error)"=w1446, "str_Level"="0", "str_Color"=w1447) -> ("error out"=w1461:errorcluster)  [unwired: 6 in, 2 out]
                              n735 = call "AndorAcqSingleImgToTiffStack.vi"("Image Nr"=w1459, "Total Images"=w1460, "error in (no error)"=w1461, "Exposure"=w1458, "Image Name"=w1457, "TiffHandle IN"=w1456) -> ("error out"=w1453:errorcluster, "Image"=w1455:T8, "TiffOut"=w1454:refnum<k24>)  [unwired: 3 in]
                              n736 = call "Set Shutter Status Extended.vi"("VISA Resource Name"=w1443, "Shutter Status (0: Open)"=enum16{"Open", "Close"}."Close", "error in (no error)"=w1453) -> ("VISA Resource Name Out"=w1452:refnum<visa-resource-name>, "error out"=w1442:errorcluster)  [unwired: 11 in]
                            }
                          }
                          n737 = local read "ProgramStop"() -> (w1396:bool)
                        }
                        n738 = local read "ProgramStop"() -> (w1364:bool)
                      }
                      n739 = call "tiffClose.vi"("Tiff in"=w1348) -> ("FileName"=w1350:string)  [unwired: 10 in]
                      n740 = local write "ANDORImage"(w1349) -> ()
                      n741 = String To Path(string=w1350) -> (path=w1351:path)
                      n742 = Strip Path(path=w1351) -> (name=w1352:string)  [unwired: 1 out]
                      n743 = local write "ANDORImgName"(w1352) -> ()
                    }
                    frame "INCUBATE" {
                      n744 = Multiply(x=w1476, y=1000.0) -> (x*y=w1475:dbl)
                      n745 = property on="ProgramStatusInfo" class="Str"(error in=w1473, "Value"="Incubation" ("Info")) -> (error out=w1470:errorcluster)  [unwired: 1 in, 1 out]
                      n746 = Wait (ms)(milliseconds to wait=w1475) -> ()  [unwired: 1 out]
                    }
                    frame "CHANGEREAGENT" {
                      n747 = local read "LINX Resource"() -> (w1493:T1)
                      n748 = property on="ProgramStatusInfo" class="Str"(error in=w1496, "Value"="Starting ChangeReagent" ("Info")) -> (error out=w1486:errorcluster)  [unwired: 1 in, 1 out]
                      n749 = call "ArdnoFlush.vi"("Open?"=TRUE, "error in (no error)"=w1486, "Single / Multivalve?"=FALSE, "Channel"=w1491, "LINX Resource"=w1493) -> ("error out"=w1495:errorcluster, "LINX Resource out"=w1494:T1)  [unwired: 5 in]
                      n750 = Multiply(x=w1489, y=1000.0 ("Time")) -> (x*y=w1483:dbl)
                      n751 = Wait (ms)(milliseconds to wait=w1483) -> ()  [unwired: 1 out]
                      n752 = call "ArdnoFlush.vi"("Open?"=FALSE, "error in (no error)"=w1495, "Single / Multivalve?"=TRUE, "Channel"=w1491, "LINX Resource"=w1494) -> ("error out"=w1479:errorcluster, "LINX Resource out"=w1481:T1)  [unwired: 5 in]
                      n753 = local write "LINX Resource"(w1481) -> ()
                      n754 = property on="ProgramStatusInfo" class="Str"(error in=w1479, "Value"="Finished ChangeReagent" ("Info")) -> (error out=w1492:errorcluster)  [unwired: 1 in, 1 out]
                    }
                    frame Default {
                      # "Switch for Queue Element (==Program Steps)"
                    }
                    frame "FEED" {
                      # "Number of Pump Cycles"
                      n755 = local read "CalibPumpCycleRefreshRatio"() -> (w1514:dbl)
                      n756 = property on="ProgramStatusInfo" class="Str"(error in=w1505, "Value"="Starting Feed" ("Info")) -> (error out=w1506:errorcluster)  [unwired: 1 in, 1 out]
                      n757 = Divide(x=w1507, y=w1514) -> (x/y=w1511:dbl)
                      n758 = Round Toward +Infinity(x=w1511) -> (ceil(x): smallest int >= x=w1509:dbl)
                      n759 = local read "LINX Resource"() -> (w1518:T1)
                      n760 = To Long Integer(number=w1509) -> (32bit integer=w1510:i32)
                      n761 = call "ArdnoFeed.vi"("LINX Resource"=w1518, "Single / Multiring?"=FALSE, "Channel"=u32 1, "Ring"=u16 1, "Feed Cycles"=w1510, "error in (no error)"=w1506, "All Rings"=TRUE, "Frequency"=u32 8) -> ("LINX Resource out"=w1516:T1, "error out"=w1502:errorcluster)  [unwired: 5 in, 1 out]
                      n762 = local write "LINX Resource"(w1516) -> ()
                      n763 = property on="ProgramStatusInfo" class="Str"(error in=w1502, "Value"="Finished Feed" ("Info")) -> (error out=w1501:errorcluster)  [unwired: 1 in, 1 out]
                    }
                    frame "PUMP" {
                      n764 = local read "LINX Resource"() -> (w1530:T1)
                      n765 = property on="ProgramStatusInfo" class="Str"(error in=w1529, "Value"="Starting Pump" ("Info")) -> (error out=w1523:errorcluster)  [unwired: 1 in, 1 out]
                      n766 = while {
                        tunnel: w1526 -> [w1543]
                        shift-right: [w1545] -> w1531
                        shift-left: w1530 -> [w1544]
                        tunnel: w1521 -> [w1533]
                        shift-right: [w1541] -> w1528
                        shift-left: w1523 -> [w1540]
                        shift-right: [w1535] -> _
                        shift-left: u32 0 ("millisecond timer value") -> [w1534]
                        stop <- w1539 stop-if-true
                        n767 = Greater Or Equal?(x=w1534, y=w1533) -> (x >= y?=w1532:bool)
                        n768 = Tick Count (ms)() -> (millisecond timer value=w1536:u32)
                        n769 = local read "ProgramStop"() -> (w1538:bool)
                        n770 = Add(x=w1536, y=w1534) -> (x+y=w1535:u32)
                        n771 = call "ArdnoPump.vi"("LINX Resource"=w1544, "Pump Cycles"=1, "Pump Frequency"=w1543, "error in (no error)"=w1540, "Single/\nMultiring?"=FALSE ("Single/\nMultiring?")) -> ("LINX Resource out"=w1545:T1, "error out"=w1541:errorcluster)  [unwired: 1 out]
                        n772 = Or(x=w1532, y=w1538) -> (x .or. y?=w1539:bool)
                      }
                      n773 = local write "LINX Resource"(w1531) -> ()
                      n774 = property on="ProgramStatusInfo" class="Str"(error in=w1528, "Value"="Finished Pump" ("Info")) -> (error out=w1525:errorcluster)  [unwired: 1 in, 1 out]
                    }
                  }
                }
              }
            }
          }
        }
        n775 = local read "ProgramStop"() -> (w115:bool)
      }
    }
    frame #4 {
      w1624 = u32 20002  # DRV Return Success
      n776 = local read "CalibTiffHandle"() -> (w1601:refnum<k24>)
      n777 = call "Shut Down.vi"() -> ("function return"=w1622:u32)  [unwired: 10 in, 1 out]
      n778 = Not Equal?(x=w1624, y=w1622) -> (x != y?=w1623:bool)
      n779 = case shown="True" w1623 {
        tunnel: w1622 -> [_ w1633]
        tunnel: [errorcluster {"status"=FALSE, "code"=0, "source"=""} ("error constant") w1628] -> w1610
        frame False {
        }
        frame True {
          n780 = call "AndorConvertErrCodeToMessage.vi"("function return"=w1633) -> ("Element Return"=w1632:cluster{i32, string})  [unwired: 10 in]
          n781 = Unbundle(w1632) -> (w1630:i32, w1631:string)
          n782 = Bundle By Name(cluster=errorcluster {"status"=FALSE, "code"=0, "source"=""} ("error constant"), "status"=TRUE, "code"=w1630, "source"=w1631) -> (w1628:errorcluster)
        }
      }
      n783 = Not A Number/Path/Refnum?(number/path/refnum=w1601) -> (NaN/Path/Refnum?=w1602:bool)
      n784 = local read "IX 81 Port"() -> (w1615:refnum<visa-resource-name>)
      n785 = case shown="False" w1602 {
        tunnel: w1601 -> [w1625 _]
        frame False {
          n786 = call "tiffClose.vi"("Tiff in"=w1625) -> ()  [unwired: 10 in, 1 out]
        }
        frame True {
        }
      }
      n787 = call "Logout Device.vi"("Device Number (1)"=1, "VISA Resource Name"=w1615) -> ("error out"=w1616:errorcluster, "VISA Resource Name Out"=w1620:refnum<visa-resource-name>)  [unwired: 8 in]
      n788 = local read "LINX Resource"() -> (w1608:T1)
      n789 = local read "TANGO"() -> (w1604:i32)
      n790 = local read "SOLA"() -> (w1611:u32)
      n791 = call "Logout Device.vi"("error in (no error)"=w1616, "Device Number (1)"=2, "VISA Resource Name"=w1620) -> ("error out"=w1617:errorcluster, "VISA Resource Name Out"=w1621:refnum<visa-resource-name>)  [unwired: 7 in]
      n792 = call "ArdnoAllValvesClosed.vi"("LINX Resource"=w1608) -> ("error out"=w1606:errorcluster, "LINX Resource out"=w1607:T1)  [unwired: 9 in]
      n793 = call <vilib>:"Close.vi"("VISA Resource Name"=w1621, "error in (no error)"=w1617) -> ("error out"=w1614:errorcluster)  [unwired: 13 in]
      n794 = call <vilib>:"Close.vi"("Error In"=w1606, "LINX Resource"=w1607) -> ("Error Out"=w1613:errorcluster)  [unwired: 9 in]
      n795 = call "lm Shut Down.vi"("hSerial"=w1611) -> ("error out"=w1612:errorcluster)  [unwired: 9 in, 1 out]
      n796 = call "Disconnect.vi"("lLSID"=w1604) -> ("error out"=w1605:errorcluster)  [unwired: 1 in]
      n797 = Merge Errors(w1609, w1614, w1613, w1612, w1605, w1610) -> (w1603:errorcluster)
    }
  }
  n798 = property on="Pane" class="Pane"() -> (error out=w16:errorcluster, "Controls[]"=w18:refnum<vi>[])  [unwired: 2 in, 1 out]
  n799 = control-ref of="This VI"() -> (w17:refnum<vi>)
  n800 = for {
    tunnel: w18 -> [w1637] mode=indexing
    shift-right: [w1634] -> w13
    shift-left: w16 -> [w1635]
    n801 = property class="Ctl"(reference=w1637, error in=w1635, "DisabledEnum"=T9."Enabled" ("Disabled")) -> (error out=w1634:errorcluster)  [unwired: 1 out]
  }
  n802 = invoke class="VI" method="Default Vals.Reinit All"(reference=w17) -> (error out=w15:errorcluster)  [unwired: 2 in, 2 out]
  n803 = property on="ProgramStop" class="Bool (strict)"("Value"=FALSE ("ProgramStop")) -> (error out=w10:errorcluster)  [unwired: 2 in, 1 out]
  n804 = Merge Errors(w13, w15, w12, w10) -> (→"error out":errorcluster)
